vi "Dashboard Main.vi"() -> ()   [LabVIEW 2019]
uses:
  2021-MARS-Swerve/Subsystems/Drive/Drive_Orientation_States.ctl
  <vilib>/Utility/miscctls.llb/LVRowAndColumnTypeDef.ctl
  <vilib>/event_ctls.llb/eventvkey.ctl
  77231be5-4dfd-47d5-a2ff-3724d3268e1c.vi
  6c3be22e-c06e-40dd-b218-0ec3cd26438d.vi
  2be0e37a-cf1f-4fec-827e-dc22e69ce85b.vi
  b3ffd77c-c7a0-4f90-8868-8b56e10d7f8c.vi
  67fa5a46-adf3-4589-a2f7-66a250c43ad7.vi
  788908d1-300c-4db3-916d-f2facaeaae96.vi
  e87f41cb-5a92-4aba-b85e-f5fa50e1b7bd.vi
  bca209f3-dc8a-45d9-88b4-0d3b0861506d.vi
  fb4473b5-3a86-49a6-a9b5-0e1129129e81.vi
  849cc23d-0ef3-4264-9ef7-306e991d33d4.vi
  16c4a620-4255-445b-bb5a-a821105b922f.vi
  55761e46-cf36-4bf9-9854-b902932db1d3.vi
  <vilib>/Rock Robotics/Network Tables/NT Write Boolean.vi
  <vilib>/Rock Robotics/Network Tables/NT Read Boolean.vi
  MARS Created VIs/GlobalDataNames.vi
  <vilib>/Rock Robotics/Network Tables/NT Read Boolean Array.vi
  <vilib>/Rock Robotics/Network Tables/NT Read Numeric Array.vi
  <vilib>/Rock Robotics/Network Tables/NT Write Boolean Array.vi
  <vilib>/Rock Robotics/Network Tables/NT Write String Array.vi
  <vilib>/Rock Robotics/Network Tables/NT Write Numeric Array.vi
  <vilib>/Rock Robotics/WPI/Dashboard/WPI_DashboardLogging Global.vi
  <vilib>/Utility/Data Type/NI_Data Type.lvlib
  <vilib>/Utility/Data Type/Type Definitions/Data Type.ctl
panel:
  in  "Rec Mode":enum32{"Stop", "Record", "Playback"}(radio)
  in  "Camera Name Right":string(combo)="No Camera Selection"
  in  "Camera Settings Right":T1={"Frame Rate"=15, "Compression"=30, "Size"=1, "DB Camera Config"=FALSE} {"Frame Rate" scale=1.0..30.0; "Compression" scale=100.0..-1.0; "Size" items=["640x480", "320x240", "160x120"]}
  out "Driver Controls":string="pilot-\nleft joystick X & Y axes- strafe / lateral and vertical throttle\nright joystick X axis- rotational throttle\nX button- toggle between robot- and field-oriented control modes\nright bumper- auto-target\nLB- outtake\nLT- intake (toggle)\nRT- fire + flywheel spin-up\nA- Zero Drive IMU\nD-pad North: Manual Magazine Forward\nD-pad South: Manual Magazine Backward\nView Button (Left): Manual Cowl Up\nMenu Button (Right): Manual Cowl Down\n\ncopilot-\nright joystick X axis- manual turret control\nX button: Zero Turret Spin\n"
  in  "TCP":refnum<k5>
  out "Robot IP":string="0.0.0.0"
  out "Image Message":string="Timeout in Camera Communications"
  in  "Dashboard Tab":T2(tab)=enum."Operation"
  in  "Max_Ground_Speed(ft/s)":dbl
  in  "Cowl_Kp":dbl=0.06
  in  "Manual_Magazine_Power":dbl=0.4
  in  "Magazine_Firing_Throttle":dbl=0.6
  in  "Intake_Speed (%vbus)":dbl=1.0
  in  "Flywheel_Speed_Multiplier":dbl=1.0
  in  "Flywheel_Acceptable_Error":dbl=200.0
  in  "Turret_Upper_Limit":dbl=160.0
  in  "Turret_Lower_Limit":dbl=-160.0
  in  "Turret_Kd":dbl=0.001
  in  "Turret_Ki":dbl=1e-05
  in  "Turret_Kp":dbl=0.06
  in  "BL_Min Output":dbl=-0.5 min=0.0
  in  "BR_Max Ouput":dbl=0.5 min=0.0
  in  "BR_Int Error Window":dbl=20.0 min=0.0
  in  "BR_N-Int":i32=10 min=0
  in  "BR_N-Diff":i32=10 min=0
  in  "BR_Kd":dbl min=0.0
  in  "BR_Ki":dbl min=0.0
  in  "BR_Kp":dbl=0.0028 min=0.0
  in  "BL_Min Output":dbl=-0.5 min=0.0
  in  "BL_Max Ouput":dbl=0.5 min=0.0
  in  "BL_Int Error Window":dbl=20.0 min=0.0
  in  "BL_N-Int":i32=10 min=0
  in  "BL_N-Diff":i32=10 min=0
  in  "BL_Kd":dbl min=0.0
  in  "BL_Ki":dbl min=0.0
  in  "BL_Kp":dbl=0.0028 min=0.0
  in  "FL_Min Output":dbl=-0.5 min=0.0
  in  "FL_Max Ouput":dbl=0.5 min=0.0
  in  "FL_Int Error Window":dbl=20.0 min=0.0
  in  "FL_N-Int":i32=10 caption="FR_N-Int" min=0
  in  "FL_N-Diff":i32=10 min=0
  in  "FL_Kd":dbl min=0.0
  in  "FL_Ki":dbl min=0.0
  in  "FL_Kp":dbl=0.0028 min=0.0
  in  "FR_Min Output":dbl=-0.5 min=0.0
  in  "FR_Max Ouput":dbl=0.5 min=0.0
  in  "FR_Int Error Window":dbl=20.0 min=0.0
  in  "FR_N-Int":i32=10 min=0
  in  "FR_N-Diff":i32=10 min=0
  in  "FR_Kd":dbl min=0.0
  in  "FR_Ki":dbl min=0.0
  in  "FR_Kp":dbl=0.0028 min=0.0
  in  "Auto_Play_Selector":string(combo)="Play 1"
  out "Cowl_Position(Degrees)":dbl(knob)=45.0 scale=-180.0..180.0
  out "Flywheel_Spun_Up":bool
  out "Turret_Auto_Targetted":bool
  out "Orientation_State":T3
  out "Back_Right_Drive_Command":dbl(slide) scale=0.0..1.0 scale format="%.2f"
  out "Back_Right_Angle_Command(deg)":dbl(knob) scale=180.0..-180.0 scale format="%#_6f"
  out "Back_Left_Drive_Command":dbl(slide) scale=0.0..1.0 scale format="%.2f"
  out "Back_Left_Angle_Command(deg)":dbl(knob) scale=180.0..-180.0 scale format="%#_6f"
  out "Front_Left_Drive_Command":dbl(slide) scale=0.0..1.0 scale format="%.2f"
  out "Front_Left_Angle_Command(deg)":dbl(knob) scale=180.0..-180.0 scale format="%#_6f"
  out "Front_Right_Drive_Command":dbl(slide) scale=0.0..1.0 scale format="%.2f"
  out "Front_Right_Angle_Command(deg)":dbl(knob) scale=180.0..-180.0 scale format="%#_6f"
  out "Flywheel_Velocity(RPM)":dbl(slide)=2614.0 scale=0.0..5000.0 scale format="%#_5g"
  out "Turret_Absolute_Position(Degrees)":dbl(knob)=45.0 scale=-180.0..180.0
  out "Camera Image":T4(plugin-control)
  in  "Camera Name":string(combo)="No Camera Selection"
  in  "Camera Settings":T1={"Frame Rate"=15, "Compression"=30, "Size"=1, "DB Camera Config"=TRUE} {"Frame Rate" scale=1.0..30.0; "Compression" scale=100.0..-1.0; "Size" items=["640x480", "320x240", "160x120"]}
  out "Camera Perf":string="                          "
  out "BoolTableSize":i32
  out "NumTableSize":i32
  out "StrTableSize":i32
  out "Selector":string="Initialize"
  out "NTEmpty":bool=TRUE
  out "disconnected":bool=TRUE
  out "ValuesGotOverwritten":bool
  in  "Select Auto":string(combo)="Select Autonomous ..."
  out "NT Connection":bool
  out "JS1 Z":dbl(slide) scale=-1.0..1.0 scale format="%#_2e"
  out "JS1 Graph":cluster{"X":dbl, "Y":dbl}[](graph)
  out "JS1 Buttons":T5
  out "JS2 Z":dbl(slide) scale=-1.0..1.0 scale format="%#_2e"
  out "JS2 Graph":cluster{"X":dbl, "Y":dbl}[](graph)
  out "JS2 Buttons":T5
  out "Mode":T6(ring)=enum."Disconnected"
  out "Right Camera Perf":cluster{"Bandwidth (Mbps)":dbl, "FPS":dbl}
  out "Camera Image Right":T4(plugin-control)
  in  "DB/String 9":string
  in  "DB/String 8":string
  in  "DB/String 7":string
  in  "DB/String 6":string
  in  "DB/String 5":string
  in  "DB/String 4":string
  in  "DB/String 3":string
  in  "DB/String 2":string
  in  "DB/String 1":string
  in  "DB/String 0":string
  in  "DB/Slider 0":dbl(slide) scale=0.0..5.0
  in  "DB/Slider 1":dbl(slide) scale=0.0..5.0
  in  "DB/Slider 2":dbl(slide) scale=0.0..5.0
  in  "DB/Slider 3":dbl(slide) scale=0.0..5.0
  out "DB/LED 3":bool
  out "DB/LED 2":bool
  out "DB/LED 1":bool
  out "DB/LED 0":bool
  in  "DB/Button 3":bool
  in  "DB/Button 2":bool
  in  "DB/Button 1":bool
  in  "DB/Button 0":bool caption="New Name"
  in  "Test Slider":dbl(slide) scale=0.0..100.0 scale format="%#_3g"
  in  "On/Off":bool caption="Solenoid"
  in  "Test Name":u16(ring) items=["Select the test to run..."]
  in  "Test Tree":string(tree)
  in  "Motor":cluster{"Value":dbl, "Enable":bool} {"Value" scale=-1.0..1.0 scale format="%#_3g"}
  out "Progress":T7 {"Test Progress" scale=0.0..100.0}
  in  "Rev/Fwd":cluster{"Forward":bool, "Reverse":bool}
  in  "Test Ring":u16(ring) items=["Monochrome", "Color"]
  out "Cmd Status":string
  in  "Execute Command":bool
  in  "Command Params":string[][](table)
  in  "Command Selection":i32(listbox)
  in  "CheckList":i32(listbox)
  out "Tree":string(tree)
  out "Background":bool
  # "HW"
  # "Cowl"
  # "Constant"
  # "Turret"
  # "Flywheel"
  # "Intake"
  # "Drive"
  # "Magazine"
  # "Drive Commands"
  # "Front_Left"
  # "Front_Right"
  # "Back_Left"
  # "Back_Right"
  # "HW"
  # "Joysticks"
  # "Drive Motors"
  # "Front"
  # "Right"
  # "Left"
  # "Back"
  # "This tab is a great place for autonomous settings and robot-specific values.\nPlace controls and indicators inside this tab and match name to\nDashboard Variables on robot. You can also delete this comment."
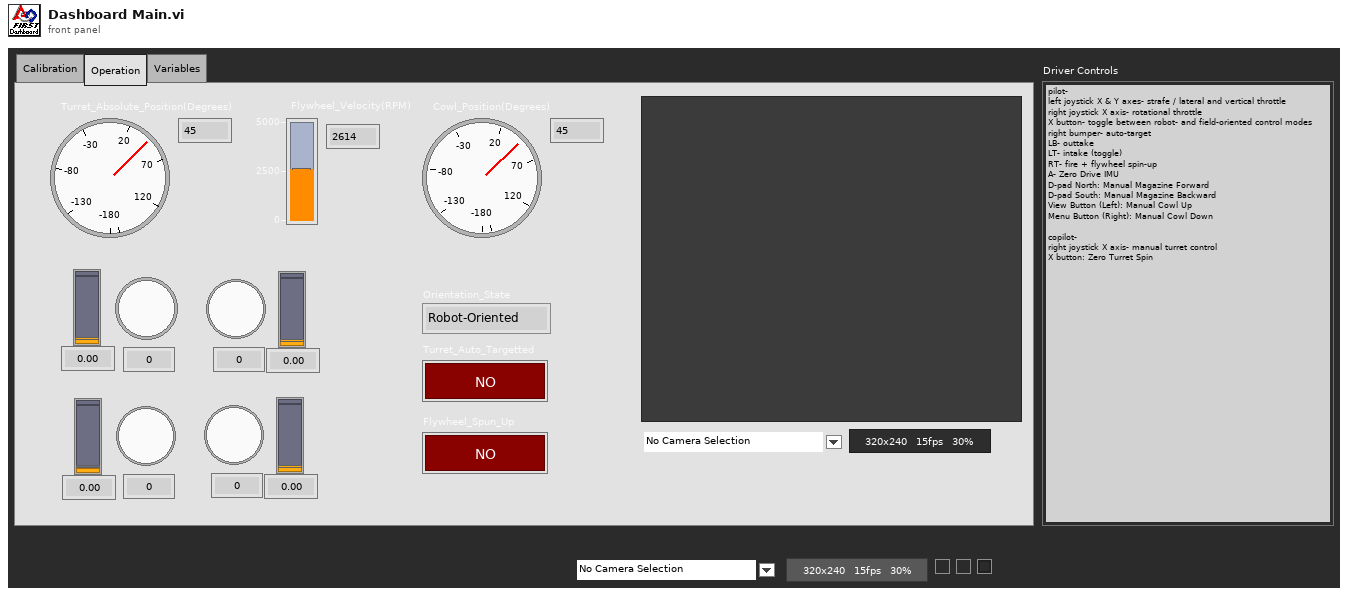
[diagram p1: front panel]
types:
  T1 = cluster{"Frame Rate":i32, "Compression":i32, "Size":u16, "DB Camera Config":bool}
  T2 = enum32{"Calibration", "Operation", "Testing", "Drive", "Camera", "Basic", "Custom", "Test", "Commands", "Checklist", "Variables"}
  T3 = typedef "Drive_Orientation_States.ctl" = enum16{"Robot-Oriented", "Field-Oriented"}
  T4 = typedef "IMAQ Image.ctl" = refnum<image>
  T5 = cluster{bool, bool, bool, bool, bool, bool, bool, bool, bool, bool, bool, bool}
  T6 = enum8{"Tele-Op Disabled", "Tele-Op Enabled", "Auto Disabled", "Auto Enabled", "Test Disabled", "Test Enabled", "Disconnected", "No Code", "E-Stop"}
  T7 = cluster{"Test Progress":u8, "Test Progress Text":string}
  T8 = cluster{"Save Path":path, "Interval (s)":dbl, "Keep":i32}
  T9 = enum32{"Drive", "Camera", "Basic", "Custom", "Test", "Commands", "Checklist", "Variables"}
  T10 = typedef "Image Type" = u32
  T11 = cluster{"IDs":cluster{"RPC field ID":u16, "Unique ID":u16}, "String":string}
  T12 = cluster{"Error Strings":string, "Disable Counts":cluster{u16, u16}, "Rail Faults":cluster{u16, u16, u16}, "Robot IP":string, "DB Mode":u8, "Event Info":cluster{"Name":string, "Type":u8, "Number":u16, "Replay":u8}}
  T13 = cluster{"Storage":cluster{"Disk Free":u64, "RAM Block":u32, "RAM free":u32}, "CPU Utilization":cluster{"CPU % ISR":sgl, "CPU % Time Crit":sgl, "CPU % Timed Str":sgl, "CPU % High":sgl, "CPU % Above":sgl, "CPU % Normal":sgl, "CPU % Low":sgl}, "CAN":cluster{"% Bus Utilization":sgl, "Bus Off Cnt":u32, "TX_FIFO Full Cnt":u32, "Receive Error Cnt":u8, "Transmit Error Cnt":u8}, "HID":cluster{"HID Outputs":u32, "Rumble Low":u16, "Rumble High":u16}[]}
  T14 = cluster{"Status bits":cluster{"Test Mode":bool, "Autonomous":bool, "Enabled":bool, "Code Start":bool, "Brownout":bool, "Reserved 2":bool, "Reserved 3":bool, "E-Stop":bool}, "Code Trace":cluster{"Disabled":bool, "TeleOp":bool, "Auto":bool, "Test":bool}, "Controller Type":enum16{"unknown", "cRIO", "roboRio"}, "Code?":enum16{"unknown", "noCode", "code"}, "Battery V":dbl}
  T15 = cluster{"Control Bits":cluster{"TestMode":bool, "Autonomous":bool, "Enabled":bool, "FMS Present":bool, bool, bool, bool, "E-Stop":bool}, "Team Station ":u8, "Countdown":sgl, "Joystick Values":cluster{"Axes":dbl[], "Buttons":bool[], "POVs":i16[]}[]}
  T16 = cluster{"Axes":dbl[], "Buttons":bool[], "POVs":i16[]}[]
  T17 = cluster{"Axes":dbl[], "Buttons":bool[], "POVs":i16[]}
  T18 = cluster{"Buttons[0]":bool, "Buttons[1]":bool, "Buttons[2]":bool, "Buttons[3]":bool, "Buttons[4]":bool, "Buttons[5]":bool, "Buttons[6]":bool, "Buttons[7]":bool, "Buttons[8]":bool, "Buttons[9]":bool, "Buttons[10]":bool, "Buttons[11]":bool}
  T19 = cluster{"Camera Image":refnum<vi>, "Dashboard Tab":refnum<vi>, "Background":refnum<vi>, "Rec Mode":refnum<vi>, "Test Slider":refnum<vi>, "On/Off ":refnum<vi>, "Test Ring":refnum<vi>, "Rev/Fwd":refnum<vi>, "Test Name":refnum<vi>, "Motor":refnum<vi>, "Progress":refnum<vi>, "CheckList":refnum<vi>, "Tree":refnum<vi>, "Test Tree":refnum<vi>, "Command Params":refnum<vi>, "Command Selection":refnum<vi>, "Execute Command":refnum<vi>, "Cmd Status":refnum<vi>, "Camera Settings":refnum<vi>, "Camera Name":refnum<vi>, "Camera Perf":refnum<vi>, "Camera Settings Right":refnum<vi>, "Camera Name Right":refnum<vi>, "Camera Image Right":refnum<vi>}
  T20 = cluster{"Global Rectangle":i32[], "Contours":cluster{"Contour Type":u32, "ROI Type":u32, "Points":i32[]}[]}
  T21 = cluster{"Camera Name":string, string, "Saved DB Images Info":cluster{"Save Path":path, "Interval (s)":dbl, "Keep":i32}}
  T22 = cluster{"Camera Name Right":string, string, "Saved DB Images Info":cluster{"Save Path":path, "Interval (s)":dbl, "Keep":i32}}
  T23 = cluster{"Operation":enum16{"Update", "Clear"}, "Color Box":u32}[]
  T24 = typedef "eventvkey.ctl" = enum16{"ASCII", "Enter", "Return", "Shift", "Ctrl", "Alt", "Cmd", "Opt", "Caps", "NumLock", "Clear", "Break", "Up", "Down", "Left", "Right", "Insert", "Delete", "Home", "End", "PageUp", "PageDown", "Escape", "Help", "Pause", "ScrollLock", "F1", "F2", "F3", "F4", "F5", "F6", "F7", "F8", "F9", "F10", "F11", "F12", "F13", "F14", "F15", "F16", "F17", "F18", "F19", "F20", "F21", "F22", "F23", "F24", "Play", "VolumeUp", "VolumeDown", "Mute", "Two Byte Char"}
  T25 = cluster{"Image Size":bool, "Image Type":bool, "Pixel Value":bool, "ROI Information":bool, "Zoom Factor":bool}
  T26 = cluster{"Operation":enum16{"Update", "Clear"}, "Color Box":u32}
  T27 = typedef "LVRowAndColumnTypeDef.ctl" = cluster{"Row":i32, "Column":i32}
  T28 = cluster{"Shift":bool, "Ctrl":bool, "Alt":bool, "Cmd":bool, "Opt":bool}
  T29 = typedef "NI_Data Type.lvlib/Data Type.ctl" = enum8{"Invalid Type", "Void", "I8", "I16", "I32", "I64", "U8", "U16", "U32", "U64", "Single Float", "Double Float", "Extended Float", "Single Complex", "Double Complex", "Extended Complex", "Enum U8", "Enum U16", "Enum U32", "Enum U64", "Single Float With Unit", "Double Float With Unit", "Extended Float With Unit", "Single Complex with Unit", "Double Complex with Unit", "Extended Complex with Unit", "Boolean", "String", "Path", "Picture", "Tag", "Array", "Cluster", "Variant", "LV Variant", "Waveform", "Timestamp", "Digital Waveform", "Digital Data", "ExpressData", "Refnum", "External Data", "VI", "Poly VI", "LabVIEW Class Instance", "Fixed Point", "Set Collection", "Map Collection"}
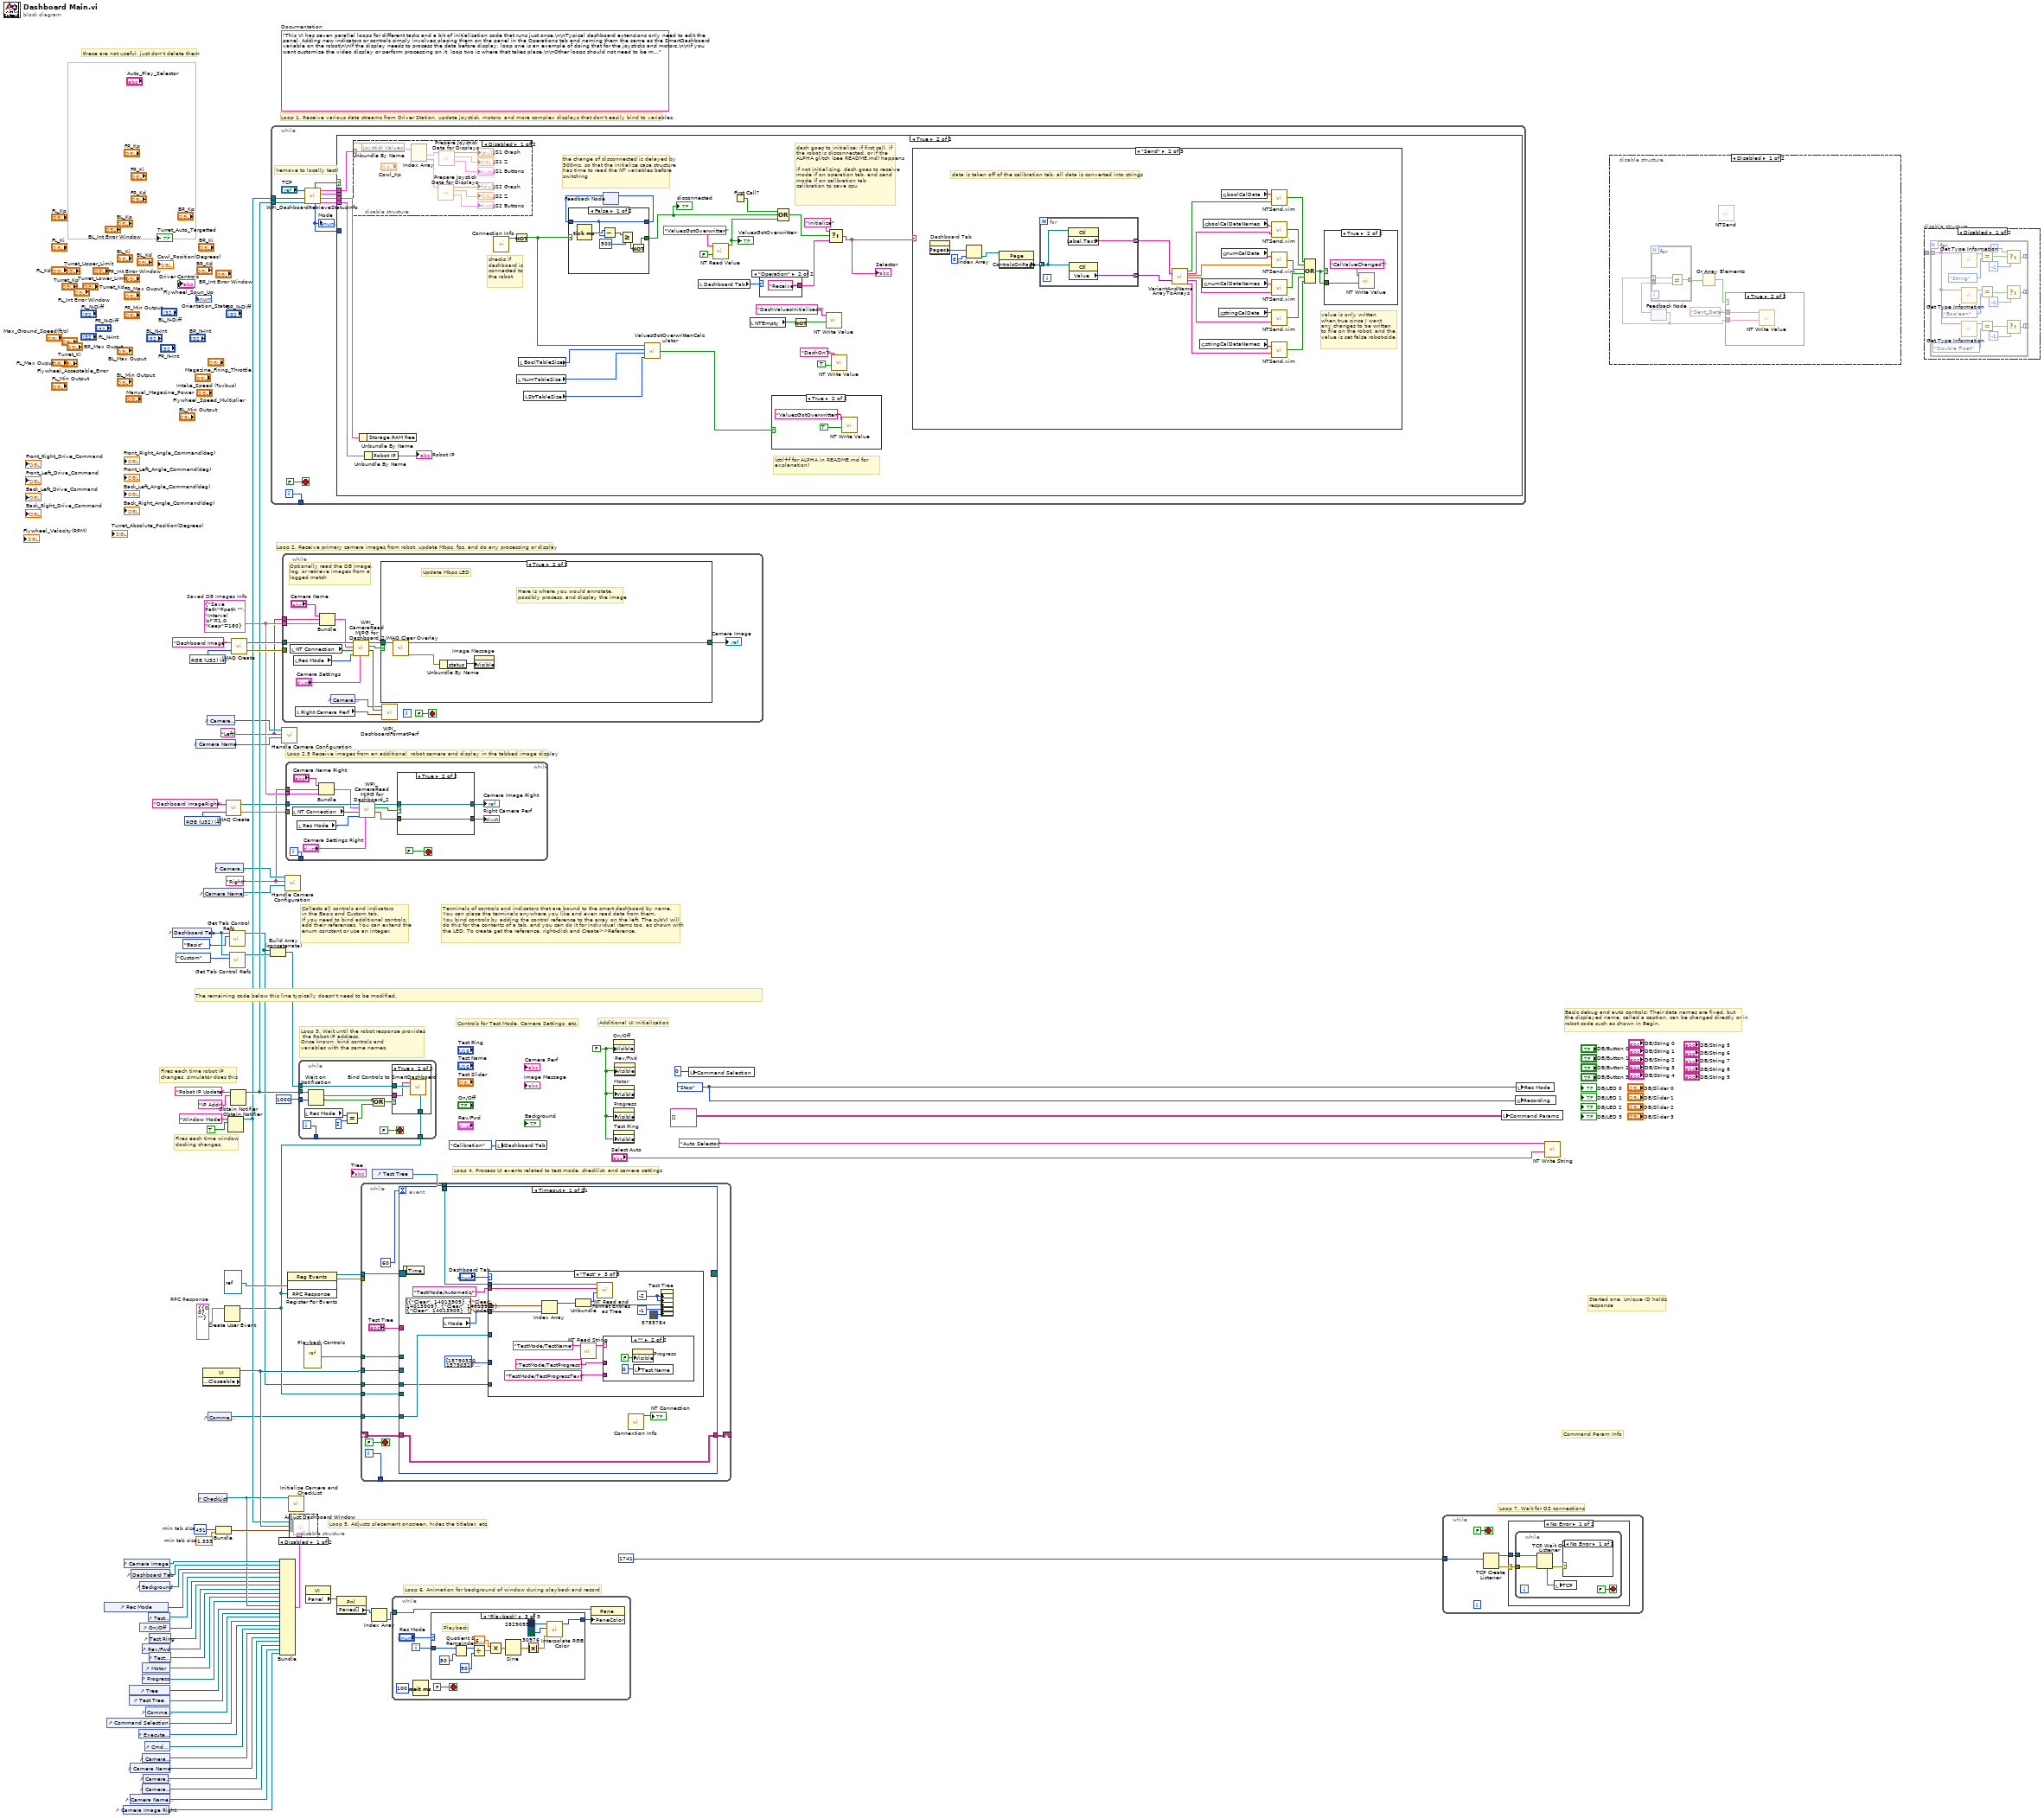
[diagram p0: block diagram]
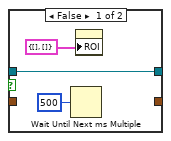
[diagram p6: hidden frame]
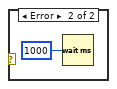
[diagram p7: hidden frame]
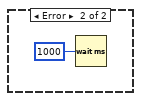
[diagram p8: hidden frame]
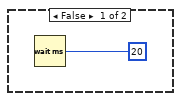
[diagram p9: hidden frame]
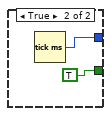
[diagram p11: hidden frame]
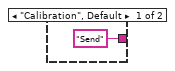
[diagram p13: hidden frame]
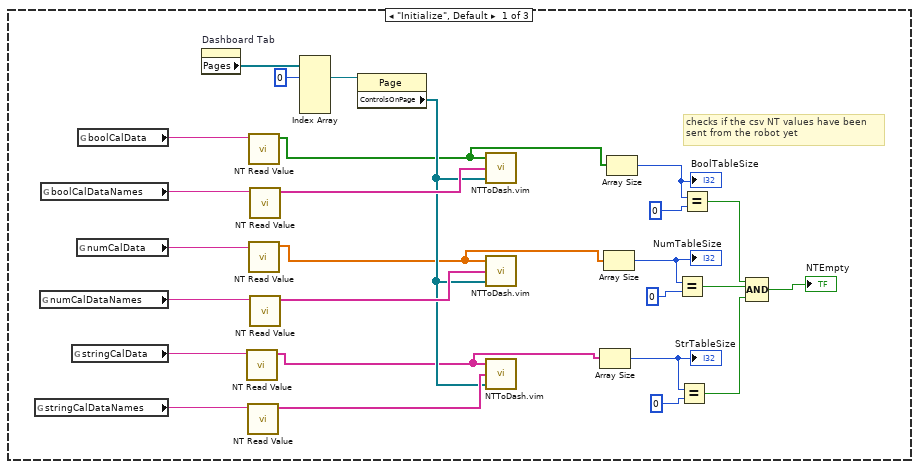
[diagram p14: hidden frame]
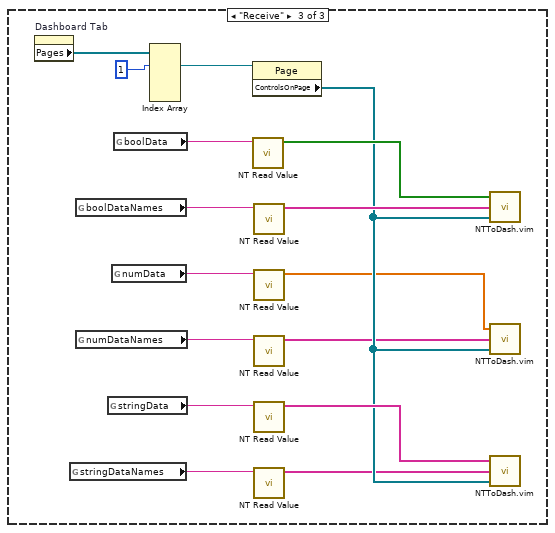
[diagram p16: hidden frame]
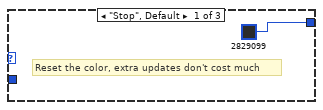
[diagram p17: hidden frame]
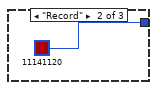
[diagram p18: hidden frame]
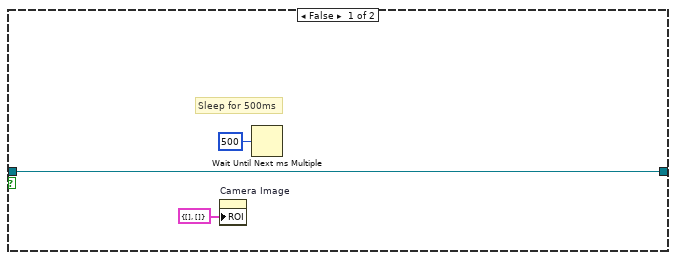
[diagram p20: hidden frame]
diagram:
  w4 = T8 {"Save Path"=path "", "Interval (s)"=1.0, "Keep"=180}  # Saved DB Images Info
  w3 = "Right"
  w2 = "Left"
  w14 = T10 4 items=["Grayscale (U8)", "Grayscale (I16)", "Grayscale (SGL)", "Complex (CSG)", "RGB (U32)", "HSL (U32)", "RGB (U64)"] ("Image Type")
  w30 = T11 {"IDs"={"RPC field ID"=0, "Unique ID"=0}, "String"=""}  # RPC Response
  w52 = 491  # min tab size
  w51 = 1.333  # min tab size
  w59 = enum32{"Stop", "Record", "Playback"}."Stop" ("Rec Mode")
  w36 = FALSE ("Visible")
  (unwired) "This VI has seven parallel loops for different tasks and a bit of initialization code that runs just once.\n\nTypical dashboard extensions only need to edit the panel. Adding new indicators or controls simply involves placing them on the panel in the Operations tab and naming them the same as the SmartDashboard variable on the robot\n\nIf the display needs to process the data before display, loop one is an example of doing that for the joysticks and motors.\n\nIf you want customize the video display or perform processing on it, loop two is where that takes place.\n\nOther loops should not need to be modified. They are pretty standard, and document the task they perform."  # Documentation
  w76 = T10 4 items=["Grayscale (U8)", "Grayscale (I16)", "Grayscale (SGL)", "Complex (CSG)", "RGB (U32)", "HSL (U32)", "RGB (U64)"] ("Image Type")
  # "these are not useful, just don't delete them"
  # "Loop 2.5 Receive images from an additional  robot camera and display in the tabbed image display"
  # "Command Param Info"
  # "Started one, Unique ID holds\nresponse"
  # "Loop 7. Wait for DS connections"
  # "Basic debug and auto controls: Their data names are fixed, but\nthe displayed name, called a caption, can be changed directly or in\nrobot code such as shown in Begin."
  # "Controls for Test Mode, Camera Settings, etc."
  # "Additional UI Initialization"
  # "Loop 6. Animation for background of window during playback and record"
  # "Fires each time robot IP\nchanges, simulator does this"
  # "Fires each time window\ndocking changes."
  # "Collects all controls and indicators\nin the Basic and Custom tab.\nIf you need to bind additional controls,\nadd their references. You can extend the\nenum constant or use an integer."
  # "The remaining code below this line typically doesn't need to be modified."
  # "Loop 4. Process UI events related to test mode, checklist, and camera settings"
  # "Terminals of controls and indicators that are bound to the smart dashboard by name.\nYou can place the terminals anywhere you like and even read data from them.\nYou bind controls by adding the control reference to the array on the left. The subVI will\ndo this for the contents of a tab, and you can do it for individual items too, as shown with\nthe LED. To create get the reference, right-click and Create>>Reference."
  # "Loop 3. Wait until the robot response provides\n the Robot IP address.\nOnce known, bind controls and\nvariables with the same names."
  # "Loop 5. Adjusts placement onscreen, hides the titlebar, etc."
  # "Loop 1. Receive various data streams from Driver Station, update joystick, motors, and more complex displays that don't easily bind to variables."
  # "Loop 2. Receive primary camera images from robot, update Mbps, fps, and do any processing or display"
  n1 = control-ref of="Rec Mode"() -> (w42:refnum<vi>)
  n2 = control-ref of="Command Selection"() -> (w29:refnum<vi>)
  n3 = control-ref of="Camera Image Right"() -> (w7:refnum<vi>)
  n4 = control-ref of="Camera Image"() -> (w54:refnum<vi>)
  n5 = control-ref of="Tree"() -> (w46:refnum<vi>)
  n6 = control-ref of="Test Tree"() -> (w45:refnum<vi>)
  n7 = control-ref of="Camera Name"() -> (w20:refnum<vi>)
  n8 = control-ref of="Camera Name Right"() -> (w8:refnum<vi>)
  n9 = control-ref of="Dashboard Tab"() -> (w53:refnum<vi>)
  n10 = control-ref of="Execute Command"() -> (w31:refnum<vi>)
  n11 = control-ref of="Background"() -> (w49:refnum<vi>)
  n12 = control-ref of="On/Off"() -> (w40:refnum<vi>)
  n13 = control-ref of="Progress"() -> (w37:refnum<vi>)
  n14 = control-ref of="Camera Settings"() -> (w21:refnum<vi>)
  n15 = control-ref of="Camera Settings Right"() -> (w9:refnum<vi>)
  n16 = control-ref of="Rev/Fwd"() -> (w38:refnum<vi>)
  n17 = control-ref of="Motor"() -> (w43:refnum<vi>)
  n18 = control-ref of="Camera Perf"() -> (w19:refnum<vi>)
  n19 = control-ref of="Cmd Status"() -> (w25:refnum<vi>)
  n20 = control-ref of="Command Params"() -> (w32:refnum<vi>)
  n21 = control-ref of="Test Slider"() -> (w41:refnum<vi>)
  n22 = control-ref of="Test Ring"() -> (w39:refnum<vi>)
  n23 = control-ref of="Test Name"() -> (w44:refnum<vi>)
  n24 = control-ref of="Dashboard Tab"() -> (w57:refnum<vi>)
  n25 = control-ref of="Camera Name"() -> (w22:refnum<vi>)
  n26 = control-ref of="CheckList"() -> (w47:refnum<vi>)
  n27 = property class="VI" props=["Front Panel.Closeable"]() -> (reference out=w58:refnum<vi>)  [unwired: 2 in, 2 out]
  n28 = control-ref of="Camera Name Right"() -> (w10:refnum<vi>)
  n29 = control-ref of="Camera Settings"() -> (w23:refnum<vi>)
  n30 = control-ref of="Command Params"() -> (w24:refnum<vi>)
  n31 = control-ref of="Camera Settings Right"() -> (w11:refnum<vi>)
  n32 = Bundle("min tab size"=w52, "min tab size"=w51) -> (w50:cluster{"min tab size":i32, "min tab size":dbl})  [unwired: 1 in]
  n33 = Create User Event(user event datatype=w30) -> (user event=w26:refnum<user-event>)  [unwired: 1 in, 1 out]
  n34 = call "IMAQ Create"("Image Name"="Dashboard ImageRight", "Image Type"=w14) -> ("New Image"=w13:T4, "error out"=w12:errorcluster)  [unwired: 2 in, 1 out]
  n35 = Obtain Notifier(name (unnamed)="Window Mode", notification data type=TRUE) -> (notifier out=w34:refnum<notifier>)  [unwired: 2 in, 2 out]
  n36 = call <vilib>:"Get Tab Control Refs.vi"("Page Index"=T9."Basic" ("Dashboard Tab"), "TabControl in"=w57) -> ("ControlsOnPage"=w18:refnum<vi>[])  [unwired: 9 in]
  n37 = call <vilib>:"Get Tab Control Refs.vi"("Page Index"=T9."Custom" ("Dashboard Tab"), "TabControl in"=w57) -> ("ControlsOnPage"=w56:refnum<vi>[])  [unwired: 9 in]
  n38 = Obtain Notifier(name (unnamed)="Robot IP Update", notification data type="IP Addr" ("name (unnamed)")) -> (notifier out=w35:refnum<notifier>)  [unwired: 2 in, 2 out]
  n39 = call "IMAQ Create"("Image Name"="Dashboard Image", "Image Type"=w76) -> ("New Image"=w74:T4, "error out"=w73:errorcluster)  [unwired: 2 in, 1 out]
  n40 = Build Array (concatenate)(w18, w56) -> (w55:refnum<vi>[])
  n41 = while {
    tunnel: [w86] -> _
    tunnel: w35 -> [w81]
    tunnel: w34 -> [w78]
    i -> [w86]
    stop <- FALSE stop-if-true
    # "(remove to locally test)"
    n42 = call <vilib>:"WPI_DashboardRetrieveStatusInfo.vi"("Binding Refnum"=w81, "Window Mode Notifier"=w78, "TCP Cnx"="TCP") -> ("Power and Errors"=w82:T12, "Robot Metrics"=w84:T13, "Status Info"=w85:T14, "Control Info"=w83:T15, "Robot Mode"=w80:T6, "Process?"=w77:bool)  [unwired: 3 in]
    "Mode" <- w80
    n43 = case shown="True" w77 {
      tunnel: w85 -> [_ _]
      tunnel: w84 -> [_ w115]
      tunnel: w83 -> [_ w114]
      tunnel: w82 -> [_ w113]
      tunnel: w80 -> [_ _]
      frame False {
        n44 = Wait (ms)(milliseconds to wait=u32 20) -> ()  [unwired: 1 out]
      }
      frame True {
        # "checks if dashboard is connected to the robot"
        # "(ctrl+f for ALPHA in README.md for explanation)"
        # "the change of disconnected is delayed by 500ms, so that the initialize case structure has time to read the NT variables before switching"
        # "dash goes to initialize: if first call, if\nthe robot is disconnected, or if the ALPHA glitch (see README.md) happens\n\nif not initializing, dash goes to receive mode if on operation tab, and send mode if on calibration tab\ncalibration to save cpu"
        n45 = disable-structure shown="Disabled" {
          disable-tunnel: w114 -> [w135 _]
          frame Disabled {
            n46 = Unbundle By Name(w135) -> ("Joystick Values"=w134:T16)
            n47 = Index Array(array=w134) -> (element #1=w133:T17, element #2=w129:T17)  [unwired: 2 in]
            n48 = call "Prepare Joystick Data for Displays.vi"("Joystick Values"=w129) -> ("Buttons"=→"JS2 Buttons":T18, "Z Axis"=→"JS2 Z":dbl, "Cartesian Data"=→"JS2 Graph":cluster{"X axis":dbl, "X axis":dbl}[])  [unwired: 8 in]
            n49 = call "Prepare Joystick Data for Displays.vi"("Joystick Values"=w133) -> ("Buttons"=→"JS1 Buttons":T18, "Z Axis"=→"JS1 Z":dbl, "Cartesian Data"=→"JS1 Graph":cluster{"X axis":dbl, "X axis":dbl}[])  [unwired: 8 in]
          }
          frame Enabled {
          }
        }
        n50 = Unbundle By Name(w115) -> ()  [unwired: 1 out]
        n51 = Unbundle By Name(w113) -> ("Robot IP"=→"Robot IP":string)
        n52 = call <vilib>:"Connection Info.vi"() -> ("Connected"=w101:bool)  [unwired: 10 in, 1 out]
        n53 = Not(x=w101) -> (.not. x?=w94:bool)
        n54 = local read "NumTableSize"() -> (w96:i32)
        n55 = local read "BoolTableSize"() -> (w97:i32)
        n56 = local read "StrTableSize"() -> (w95:i32)
        n57 = feedback #1() -> (w98:u32)  [unwired: 1 in]
        n58 = case shown="False" w94 {
          tunnel: [w118 TRUE] -> w100
          tunnel: [w122 w124] -> w99
          tunnel: w98 -> [w122 _]
          frame False {
            n59 = Tick Count (ms)() -> (millisecond timer value=w123:u32)
            n60 = Subtract(x=w123, y=w122) -> (x-y=w121:u32)
            n61 = Greater Or Equal?(x=w121, y=u32 500) -> (x >= y?=w119:bool)
            n62 = Not(x=w119) -> (.not. x?=w118:bool)
          }
          frame True {
            n63 = Tick Count (ms)() -> (millisecond timer value=w124:u32)
          }
        }
        "disconnected" <- w100
        n64 = feedback-in #1(w99) -> ()
        n65 = call "ValuesGotOverwrittenCalculator.vi"("StrTableSize"=w95, "NumTableSize"=w96, "BoolTableSize"=w97, "disconnected"=w94) -> ("ValuesGotOverwritten"=w93:bool)
        n66 = local read "Dashboard Tab"() -> (w109:T2)
        n67 = call-poly <vilib>:"NT Read Value.vi"("Default Value"=FALSE, "Name"="ValuesGotOverwritten") -> ("Boolean"=w90:bool)  [unwired: 8 in, 1 out]
        "ValuesGotOverwritten" <- w90
        n68 = First Call?() -> (First Call?: T/F=w102:bool)
        n69 = local read "NTEmpty"() -> (w104:bool)
        n70 = case shown="\"Operation\"" w109 {
          tunnel: ["Send" "Receive"] -> w108
          frame "Calibration", Default {
          }
          frame "Operation" {
          }
        }
        n71 = case shown="True" w93 {
          frame False {
          }
          frame True {
            n72 = call-poly <vilib>:"NT Write Value.vi"("Boolean"=TRUE, "Name"="ValuesGotOverwritten") -> ()  [unwired: 9 in, 1 out]
          }
        }
        n73 = Compound Arithmetic op=OR(w102, w100, w90) -> (w106:bool)
        n74 = Not(x=w104) -> (.not. x?=w103:bool)
        n75 = call-poly <vilib>:"NT Write Value.vi"("Boolean"=w103, "Name"="DashValuesInitialized?") -> ()  [unwired: 9 in, 1 out]
        n76 = Select(t="Initialize", s=w106, f=w108) -> (s? t:f=w89:string)
        "Selector" <- w89
        n77 = call-poly <vilib>:"NT Write Value.vi"("Boolean"=TRUE, "Name"="DashOn?") -> ()  [unwired: 9 in, 1 out]
        n78 = case shown="\"Send\"" w89 {
          frame "Initialize", Default {
            # "checks if the csv NT values have been\nsent from the robot yet"
            n79 = global read "GlobalDataNames.vi" "stringCalDataNames"() -> (w151:string)
            n80 = global read "GlobalDataNames.vi" "numCalDataNames"() -> (w153:string)
            n81 = global read "GlobalDataNames.vi" "boolCalDataNames"() -> (w156:string)
            n82 = global read "GlobalDataNames.vi" "stringCalData"() -> (w152:string)
            n83 = global read "GlobalDataNames.vi" "numCalData"() -> (w154:string)
            n84 = global read "GlobalDataNames.vi" "boolCalData"() -> (w155:string)
            n85 = property on="Dashboard Tab" class="TabCtl (strict)"() -> ("Pages"=w157:refnum<vi>[])  [unwired: 2 in, 2 out]
            n86 = call-poly <vilib>:"NT Read Value.vi"("Name"=w152) -> ("String Array"=w148:string[])  [unwired: 9 in, 1 out]
            n87 = call-poly <vilib>:"NT Read Value.vi"("Name"=w151) -> ("String Array"=w162:string[])  [unwired: 9 in, 1 out]
            n88 = call-poly <vilib>:"NT Read Value.vi"("Name"=w155) -> ("Boolean Array"=w150:bool[])  [unwired: 9 in, 1 out]
            n89 = call-poly <vilib>:"NT Read Value.vi"("Name"=w154) -> ("Numeric Array"=w149:dbl[])  [unwired: 9 in, 1 out]
            n90 = call-poly <vilib>:"NT Read Value.vi"("Name"=w156) -> ("String Array"=w163:string[])  [unwired: 9 in, 1 out]
            n91 = call-poly <vilib>:"NT Read Value.vi"("Name"=w153) -> ("String Array"=w161:string[])  [unwired: 9 in, 1 out]
            n92 = Index Array(array=w157, index #1=0 ("index")) -> (element #1=w160:refnum<vi>)  [unwired: 4 in, 4 out]
            n93 = property class="Page"(reference=w160) -> ("ControlsOnPage"=w158:refnum<vi>[])  [unwired: 1 in, 2 out]
            n94 = call "NTToDash.vim"("Controls on Page[]"=w158, "Names Array"=w163, "Data Array"=w150) -> ()  [unwired: 1 in]
            n95 = call "NTToDash.vim"("Controls on Page[]"=w158, "Names Array"=w161, "Data Array"=w149) -> ()  [unwired: 1 in]
            n96 = call "NTToDash.vim"("Controls on Page[]"=w158, "Names Array"=w162, "Data Array"=w148) -> ()  [unwired: 1 in]
            n97 = Array Size(array=w148) -> (size(s)=w143:i32)
            "StrTableSize" <- w143
            n98 = Array Size(array=w149) -> (size(s)=w145:i32)
            "NumTableSize" <- w145
            n99 = Array Size(array=w150) -> (size(s)=w147:i32)
            "BoolTableSize" <- w147
            n100 = Equal?(x=w145, y=0 ("size(s)")) -> (x = y?=w140:bool)
            n101 = Equal?(x=w143, y=0 ("size(s)")) -> (x = y?=w141:bool)
            n102 = Equal?(x=w147, y=0 ("size(s)")) -> (x = y?=w139:bool)
            n103 = Compound Arithmetic op=AND(w139, w140, w141) -> (→"NTEmpty":bool)
          }
          frame "Send" {
            # "value is only written\nwhen true since I want\nany changes to be written\nto file on the robot, and the \nvalue is set false robot-side"
            # "data is taken off of the calibration tab, all data is converted into strings"
            n104 = property on="Dashboard Tab" class="TabCtl (strict)"() -> ("Pages"=w188:refnum<vi>[])  [unwired: 2 in, 2 out]
            n105 = Index Array(array=w188, index=0) -> (element=w186:refnum<vi>)
            n106 = property class="Page"(reference=w186) -> ("ControlsOnPage"=w185:refnum<vi>[])  [unwired: 1 in, 2 out]
            n107 = for {
              tunnel: w185 -> [w193] mode=indexing
              tunnel: [w192] -> w184 mode=indexing
              tunnel: [w191] -> w183 mode=indexing
              n108 = property class="Ctl"(reference=w193) -> ("Label.Text"=w192:string)  [unwired: 1 in, 2 out]
              n109 = property class="Ctl"(reference=w193) -> ("Value"=w191:variant)  [unwired: 1 in, 2 out]
            }
            n110 = call "VariantAndNameArrayToArrays.vi"("Names Array"=w184, "Variant Array"=w183) -> ("bool"=w182:bool[], "boolNames"=w181:string[], "num"=w179:dbl[], "numNames"=w178:string[], "string"=w164:string[], "stringNames"=w180:string[])  [unwired: 12 in]
            n111 = global read "GlobalDataNames.vi" "stringCalDataNames"() -> (w173:string)
            n112 = global read "GlobalDataNames.vi" "numCalDataNames"() -> (w175:string)
            n113 = global read "GlobalDataNames.vi" "boolCalDataNames"() -> (w176:string)
            n114 = global read "GlobalDataNames.vi" "stringCalData"() -> (w174:string)
            n115 = global read "GlobalDataNames.vi" "numCalData"() -> (w177:string)
            n116 = global read "GlobalDataNames.vi" "boolCalData"() -> (w172:string)
            n117 = call "NTSend.vim"("Array"=w182, "name"=w172) -> ("Write?"=w171:bool)
            n118 = call "NTSend.vim"("Array"=w181, "name"=w176) -> ("Write?"=w170:bool)
            n119 = call "NTSend.vim"("Array"=w179, "name"=w177) -> ("Write?"=w169:bool)
            n120 = call "NTSend.vim"("Array"=w178, "name"=w175) -> ("Write?"=w168:bool)
            n121 = call "NTSend.vim"("Array"=w164, "name"=w174) -> ("Write?"=w167:bool)
            n122 = call "NTSend.vim"("Array"=w180, "name"=w173) -> ("Write?"=w166:bool)
            n123 = Compound Arithmetic op=OR(w171, w170, w169, w168, w167, w166) -> (w165:bool)
            n124 = case shown="True" w165 {
              tunnel: w165 -> [_ w190]
              frame False {
              }
              frame True {
                n125 = call-poly <vilib>:"NT Write Value.vi"("Boolean"=w190, "Name"="CalValueChanged?") -> ()  [unwired: 9 in, 1 out]
              }
            }
          }
          frame "Receive" {
            n126 = property on="Dashboard Tab" class="TabCtl (strict)"() -> ("Pages"=w207:refnum<vi>[])  [unwired: 2 in, 2 out]
            n127 = global read "GlobalDataNames.vi" "stringDataNames"() -> (w201:string)
            n128 = global read "GlobalDataNames.vi" "boolDataNames"() -> (w206:string)
            n129 = global read "GlobalDataNames.vi" "numDataNames"() -> (w203:string)
            n130 = global read "GlobalDataNames.vi" "stringData"() -> (w202:string)
            n131 = global read "GlobalDataNames.vi" "numData"() -> (w204:string)
            n132 = global read "GlobalDataNames.vi" "boolData"() -> (w205:string)
            n133 = Index Array(array=w207, index #1=1 ("index")) -> (element #1=w209:refnum<vi>)  [unwired: 4 in, 4 out]
            n134 = property class="Page"(reference=w209) -> ("ControlsOnPage"=w197:refnum<vi>[])  [unwired: 1 in, 2 out]
            n135 = call-poly <vilib>:"NT Read Value.vi"("Name"=w205) -> ("Boolean Array"=w200:bool[])  [unwired: 9 in, 1 out]
            n136 = call-poly <vilib>:"NT Read Value.vi"("Name"=w206) -> ("String Array"=w199:string[])  [unwired: 9 in, 1 out]
            n137 = call-poly <vilib>:"NT Read Value.vi"("Name"=w204) -> ("Numeric Array"=w195:dbl[])  [unwired: 9 in, 1 out]
            n138 = call-poly <vilib>:"NT Read Value.vi"("Name"=w203) -> ("String Array"=w194:string[])  [unwired: 9 in, 1 out]
            n139 = call-poly <vilib>:"NT Read Value.vi"("Name"=w202) -> ("String Array"=w198:string[])  [unwired: 9 in, 1 out]
            n140 = call-poly <vilib>:"NT Read Value.vi"("Name"=w201) -> ("String Array"=w196:string[])  [unwired: 9 in, 1 out]
            n141 = call "NTToDash.vim"("Controls on Page[]"=w197, "Names Array"=w199, "Data Array"=w200) -> ()  [unwired: 1 in]
            n142 = call "NTToDash.vim"("Controls on Page[]"=w197, "Names Array"=w194, "Data Array"=w195) -> ()  [unwired: 1 in]
            n143 = call "NTToDash.vim"("Controls on Page[]"=w197, "Names Array"=w196, "Data Array"=w198) -> ()  [unwired: 1 in]
          }
        }
      }
    }
  }
  n144 = Bundle("Camera Image"=w54, "Dashboard Tab"=w53, "Background"=w49, "Rec Mode"=w42, "Test Slider"=w41, "On/Off"=w40, "Test Ring"=w39, "Rev/Fwd"=w38, "Test Name"=w44, "Motor"=w43, "Progress"=w37, "CheckList"=w47, "Tree"=w46, "Test Tree"=w45, "Command Params"=w32, "Command Selection"=w29, "Execute Command"=w31, "Cmd Status"=w25, "Camera Settings"=w21, "Camera Name"=w20, "Camera Perf"=w19, "Camera Settings Right"=w9, "Camera Name Right"=w8, "Camera Image Right"=w7) -> (w48:T19)  [unwired: 1 in]
  n145 = call "Handle Camera Configuration.vi"("CameraNameRef"=w22, "Display Name"=w2, "ClusterRef"=w23) -> ()  [unwired: 9 in]
  n146 = while {
    tunnel: w74 -> [w223]
    tunnel: w73 -> [_]
    tunnel: w4 -> [w216]
    tunnel: w2 -> [w213]
    stop <- FALSE stop-if-true
    # "Optionally read the DB image,\nlog, or retrieve images from a\nlogged match"
    n147 = local read "NT Connection"() -> (w217:bool)
    n148 = local read "Rec Mode"() -> (w220:enum32{"Stop", "Record", "Playback"})
    n149 = local read "Right Camera Perf"() -> (w211:cluster{"Bandwidth (Mbps)":dbl, "FPS":dbl})
    n150 = Bundle("Camera Name"="Camera Name", w213, "Saved DB Images Info"=w216) -> (w215:T21)  [unwired: 1 in]
    n151 = control-ref of="Camera Perf"() -> (w210:refnum<vi>)
    n152 = call <vilib>:"WPI_CameraRead MJPG for Dashboard_2.vi"("Camera Settings"="Camera Settings", "Rec Mode"=w220, "NT Connection"=w217, "Capture Info"=w215, "Image in"=w223) -> ("perf info"=w212:cluster{"Bandwidth (Mbps)":dbl, "fps":dbl}, "Active"=w221:bool, "Image\\ out"=w222:T4)  [unwired: 4 in]
    n153 = case shown="True" w221 {
      tunnel: w222 -> [w226 w229]
      tunnel: [w226 w228] -> w218
      frame False {
        # "Sleep for 500ms"
        n154 = property on="Camera Image" class="ImageControl"("ROI"=T20 {"Global Rectangle"=[], "Contours"=[]}) -> ()  [unwired: 2 in, 2 out]
        n155 = Wait Until Next ms Multiple(millisecond multiple=u32 500) -> ()  [unwired: 1 out]
      }
      frame True {
        # "Here is where you would annotate,\npossibly process, and display the image"
        # "Update Mbps LED"
        n156 = call "IMAQ Clear Overlay"("Image"=w229) -> ("error out"=w230:errorcluster, "Image Out"=w228:T4)  [unwired: 2 in, 7 out]
        n157 = Unbundle By Name(w230) -> ("status"=w231:bool)
        n158 = property on="Image Message" class="Str"("Visible"=w231) -> ()  [unwired: 2 in, 2 out]
      }
    }
    "Camera Image" <- w218
    n159 = call <vilib>:"WPI_DashboardFormatPerf.vi"("Right Camera Perf"=w211, "Performance"=w212, "String in"=w210) -> ()  [unwired: 9 in]
  }
  n160 = call "Handle Camera Configuration.vi"("CameraNameRef"=w10, "Display Name"=w3, "ClusterRef"=w11) -> ()  [unwired: 9 in]
  n161 = while {
    tunnel: w13 -> [w246]
    tunnel: w12 -> [_]
    tunnel: [w241] -> _
    tunnel: w4 -> [w237]
    tunnel: w3 -> [w234]
    i -> [w241]
    stop <- FALSE stop-if-true
    n162 = local read "NT Connection"() -> (w238:bool)
    n163 = local read "Rec Mode"() -> (w245:enum32{"Stop", "Record", "Playback"})
    n164 = Bundle("Camera Name Right"="Camera Name Right", w234, "Saved DB Images Info"=w237) -> (w236:T22)  [unwired: 1 in]
    n165 = call <vilib>:"WPI_CameraRead MJPG for Dashboard_2.vi"("Camera Settings"="Camera Settings Right", "Rec Mode"=w245, "NT Connection"=w238, "Capture Info"=w236, "Image in"=w246) -> ("perf info"=w232:cluster{"Bandwidth (Mbps)":dbl, "fps":dbl}, "Active"=w240:bool, "Image\\ out"=w243:T4)  [unwired: 4 in]
    n166 = case shown="True" w240 {
      tunnel: w243 -> [w248 w251]
      tunnel: [w248 w251] -> w239
      tunnel: [_ w250] -> w233
      tunnel: w232 -> [_ w250]
      frame False {
        n167 = Wait Until Next ms Multiple(millisecond multiple=u32 500) -> ()  [unwired: 1 out]
        n168 = property on="Camera Image Right" class="ImageControl"("ROI"=T20 {"Global Rectangle"=[], "Contours"=[]}) -> ()  [unwired: 2 in, 2 out]
      }
      frame True {
      }
    }
    "Camera Image Right" <- w239
    "Right Camera Perf" <- w233
  }
  n169 = register-events(refnum<vi> refnum, w26) -> (reference out=w63:refnum<event-registration>, error out=w62:errorcluster)  [unwired: 2 in]
  n170 = call "Initialize Camera and CheckList.vi"("ListBox in"=w47) -> ()  [unwired: 11 in]
  n171 = disable-structure shown="Disabled" {
    disable-tunnel: w58 -> [w255 _]
    disable-tunnel: w50 -> [w254 _]
    disable-tunnel: w48 -> [w253 _]
    disable-tunnel: w34 -> [w252 _]
    frame Disabled {
      n172 = call "Adjust Dashboard Window.vi"("Sizing Refnums"=w253, "Size Constraints"=w254, "VI"=w255, "WIn Mode"=w252) -> ()  [unwired: 8 in]
    }
    frame Enabled {
    }
  }
  n173 = while {
    tunnel: w55 -> [w267]
    tunnel: w35 -> [w265]
    tunnel: [w263] -> _
    tunnel: u32 1000 ("milliseconds to wait") -> [w262]
    tunnel: w26 -> [w256]
    i -> [w263]
    stop <- FALSE stop-if-true
    n174 = local read "Rec Mode"() -> (w258:enum32{"Stop", "Record", "Playback"})
    n175 = Wait on Notification(notifier=w265, timeout in ms (-1)=w262) -> (notification=w264:string, timed out?=w260:bool)  [unwired: 2 in, 2 out]
    n176 = Equal?(x=w258, y=u16 2 ("Rec Mode")) -> (x = y?=w259:bool)
    n177 = Compound Arithmetic op=OR(invert w260, w259) -> (w261:bool)
    n178 = case shown="True" w261 {
      tunnel: w267 -> [_ w270]
      tunnel: w264 -> [_ w269]
      tunnel: w256 -> [_ w268]
      frame False {
      }
      frame True {
        n179 = call <vilib>:"Bind Controls to SmartDashboard.vi"("RPC ref"=w268, "Bound Control Refs"=w270, "Server IP Address"=w269) -> ()  [unwired: 9 in]
      }
    }
  }
  n180 = vi-ref "Playback Controls.vi"() -> (w64:refnum<vi>)
  n181 = property class="VI"() -> ("Panel"=w66:refnum<vi>)  [unwired: 2 in, 2 out]
  n182 = property class="Pnl"(reference=w66) -> ("Panes[]"=w67:refnum<vi>[])  [unwired: 1 in, 2 out]
  n183 = Index Array(array=w67) -> (element=w65:refnum<vi>)  [unwired: 1 in]
  n184 = control-ref of="Test Tree"() -> (w68:refnum<vi>)
  n185 = while {
    tunnel: [w280] -> _
    tunnel: w68 -> [w279]
    tunnel: w64 -> [w278]
    tunnel: w63 -> [w277]
    tunnel: w62 -> [_]
    tunnel: w58 -> [w276]
    tunnel: w26 -> [w275]
    tunnel: w24 -> [w274]
    shift-right: [w273] -> _
    shift-left: _ -> [w272]
    tunnel: w18 -> [w271]
    i -> [w280]
    stop <- FALSE stop-if-true
    n186 = event shown="[0] Timeout" {
      selector: w277 -> [_ _ _ _ _ _ _ _ _ _ _ _ _ _ _ _ _ _ _ _ _]
      dyn-events: [_ _ _ _ _ _ _ _ _ _ _ _ _ _ _ _ w540 _ _ _ _] -> _
      timeout: u32 60 ("milliseconds to wait") -> [_ _ _ _ _ _ _ _ _ _ _ _ _ _ _ _ _ _ _ _ _]
      tunnel: w279 -> [w292 _ _ _ _ _ _ _ _ _ _ _ _ _ _ _ _ _ _ _ _]
      tunnel: "Test Tree" -> [_ _ _ _ _ _ _ _ _ _ _ w507 w515 w517 w521 w529 _ _ _ _ _]
      tunnel: w278 -> [_ _ _ _ _ _ _ _ _ _ _ _ _ _ _ _ w542 _ w560 _ _]
      tunnel: w276 -> [_ _ _ _ _ _ _ _ _ _ _ _ _ _ _ _ w538 _ _ _ _]
      tunnel: w275 -> [_ _ _ _ _ _ _ _ _ _ _ _ _ _ _ _ w536 _ _ _ _]
      tunnel: w274 -> [w287 _ _ _ _ _ w458 _ _ _ _ _ _ _ _ _ _ _ _ _ _]
      tunnel: [w286 w335 w437 w442 w451 w455 w456 w465 w475 w482 w494 w506 w513 w516 w520 w528 w535 w555 w557 w561 w574] -> w273
      tunnel: w272 -> [w286 w335 w437 w442 w451 w455 w456 _ _ w482 w494 w506 w513 w516 w520 w528 w535 w555 w557 w561 w574]
      tunnel: w271 -> [w284 _ _ _ _ _ _ _ _ _ _ _ _ _ _ _ _ _ _ _ _]
      event Timeout {
        n187 = event-data() -> ()  [unwired: 1 in, 1 out]
        n188 = local read "Mode"() -> (w289:T6)
        n189 = case shown="\"Test\"" "Dashboard Tab" {
          tunnel: w292 -> [_ _ w308 _ _]
          tunnel: "TestMode/Automatic/" ("Name Pattern") -> [_ _ w307 _ _]
          tunnel: T23 [{"Operation"=enum."Clear", "Color Box"=14013909}, {"Operation"=enum."Clear", "Color Box"=14013909}, {"Operation"=enum."Clear", "Color Box"=14013909}, {"Operation"=enum."Clear", "Color Box"=14013909}, {"Operation"=enum."Update", "Color Box"=14013909}, {"Operation"=enum."Update", "Color Box"=16777215}, {"Operation"=enum."Clear", "Color Box"=14013909}, {"Operation"=enum."Clear", "Color Box"=14013909}, {"Operation"=enum."Clear", "Color Box"=14013909}] -> [_ _ w300 _ w328]
          tunnel: w289 -> [_ _ w299 _ w327]
          tunnel: u32[] [15790320, 15790320, 15790320, 15790320, 16777215, 16777215, 15790320, 15790320, 15790320] -> [_ _ _ _ w333]
          tunnel: w287 -> [_ _ _ _ w321]
          tunnel: w284 -> [_ w294 _ _ _]
          frame "Custom", Default {
          }
          frame "Basic" {
            n190 = call <vilib>:"WPI_DashboardUpdateNames.vi"("Controls on Tab"=w294) -> ()  [unwired: 11 in]
          }
          frame "Test" {
            w306 = -2 ("Active Item:Row Number")
            n191 = Index Array(array=w300, index=w299) -> (element=w301:T26)
            n192 = Unbundle(w301) -> ("Operation"=w302:enum16{"Update", "Clear"}, "Color Box"=w303:u32)
            n193 = call <vilib>:"NT Read String.vi"("Name"="TestMode/TestName") -> ("String"=w297:string)  [unwired: 9 in, 1 out]
            n194 = call <vilib>:"NT Read and Format Entries as Tree.vi"("Operation"=w302, "Name Pattern"=w307, "Tree Refnum"=w308) -> ()  [unwired: 7 in, 2 out]
            n195 = case shown="\"\"" w297 {
              tunnel: "TestMode/TestProgress" ("Name") -> [w310 _]
              tunnel: "TestMode/TestProgressText" ("Name") -> [w309 _]
              frame Default {
                n196 = call <vilib>:"NT Read Number.vi"("Name"=w310) -> ("Numeric"=w311:dbl)  [unwired: 9 in, 1 out]
                n197 = call <vilib>:"NT Read String.vi"("Name"=w309) -> ("String"=w312:string)  [unwired: 9 in, 1 out]
                n198 = Bundle("Numeric"=w311, "String"=w312) -> (→"Progress":cluster{"Numeric":dbl, "String":string})  [unwired: 1 in]
              }
              frame "" {
                n199 = property on="Progress" class="Clust (strict)"("Visible"=FALSE) -> ()  [unwired: 2 in, 2 out]
                n200 = local write "Test Name"(u16 0) -> ()
              }
            }
            n201 = property on="Test Tree" class="Tree (strict)"("Active Item Row Number"=w306, "ActiveColNum"=w306, "CellBG"=w303, "Active Item Row Number"=-1 ("Active Item:Row Number"), "CellBG"=u32 5789784 ("Color Box")) -> ()  [unwired: 2 in, 2 out]
          }
          frame "Variables" {
            w318 = string[] ["CameraPublisher", "Usage", "DB"]  # Items to initially close
            n202 = First Call?() -> (First Call?: T/F=w319:bool)
            n203 = control-ref of="Tree"() -> (w320:refnum<vi>)
            n204 = Select(t=w318, s=w319, f=string[] []) -> (s? t:f=w316:string[])
            n205 = call <vilib>:"NT Read and Format Entries as Tree.vi"("Tags to  Close"=w316, "Tree Refnum"=w320) -> ()  [unwired: 8 in, 2 out]
          }
          frame "Commands" {
            w329 = u32 5789784 ("Color Box")
            w330 = T27 {"Row"=-1, "Column"=-2} ("Active Cell:Active Cell")
            w332 = T27 {"Row"=-2, "Column"=-2} ("Active Cell:Active Cell")
            n206 = Index Array(array=w333, index=w327) -> (element=w331:u32)
            n207 = Index Array(array=w328, index=w327) -> (element=w326:T26)
            n208 = Unbundle(w326) -> ("Operation"=w325:enum16{"Update", "Clear"})  [unwired: 1 out]
            n209 = local read "Command Selection"() -> (w324:i32)
            n210 = property on="Command Selection" class="MCListbox (strict)"("ActiveCell"=w332, "CellBG"=w331, "ActiveCell"=w330, "CellBG"=w329) -> ()  [unwired: 2 in, 2 out]
            n211 = call <vilib>:"WPI_DashboardUpdate RPC Info.vi"("Operation"=w325) -> ("update"=w323:bool, "commands"=w322:string[][])  [unwired: 9 in]
            n212 = property on="Command Selection" class="MCListbox (strict)"("ItemNames"=w322) -> ()  [unwired: 2 in, 2 out]
            n213 = property on="Command Params" class="Tbl (strict)"("Active Cell"=w332, "Cell BG Color"=w331, "Active Cell"=w330, "Cell BG Color"=w329) -> ()  [unwired: 2 in, 2 out]
            n214 = call <vilib>:"WPI_DashboardUpdate Command Params.vi"("Update"=w323, "NewVal"=w324, "Commands"=w322, "Param Tbl"=w321) -> ()  [unwired: 7 in, 1 out]
          }
        }
        n215 = call <vilib>:"Connextion Info.vi"() -> ("Connected"=→"NT Connection":bool)  [unwired: 10 in, 1 out]
      }
      event "Test Tree": Value Change {
        # "Show appropriate\ncontrols"
        n216 = event-data() -> ("CtlRef"=w338:refnum<vi>, "NewVal"=w336:string)  [unwired: 1 in]
        n217 = call <vilib>:"WPI_UtilitiesGetTreeIOName.vi"("NewVal"=w336, "TreeControl in"=w338) -> ("I/O Name"=w339:string)  [unwired: 9 in]
        n218 = case shown="\"Camera\"" w339 {
          selector: w339 -> [_ w346 _ w368 w377 _]
          tunnel: w336 -> [_ _ w365 w367 _ w384]
          tunnel: cluster{string[]}[] [{["640x480", "320x240", "160x120"]}, {["Auto", "Fixed indoor", "Fixed outdoor 1", "Fixed outdoor 2", "Fixed fluorescent 1", "Fixed fluorescent 2", "Hold current"]}, {["Auto", "Flicker-free 50 Hz", "Flicker-free 60 Hz", "Hold current"]}, {["None", "Prioritize frame rate", "Prioritize image quality"]}, {["Monochrome", "Color"]}] -> [_ _ _ _ _ w383]
          frame Default {
            w341 = FALSE ("Visible")
            w340 = FALSE ("Visible")
            n219 = property on="Motor" class="Clust (strict)"("Visible"=w340) -> ()  [unwired: 2 in, 2 out]
            n220 = property on="Test Ring" class="Ring (strict)"("Visible"=w340) -> ()  [unwired: 2 in, 2 out]
            n221 = property on="Rev/Fwd" class="Clust (strict)"("Visible"=w341) -> ()  [unwired: 2 in, 2 out]
            n222 = property on="On/Off" class="Bool (strict)"("Visible"=w341) -> ()  [unwired: 2 in, 2 out]
            n223 = property on="Test Slider" class="Slide (strict)"("Visible"=w341) -> ()  [unwired: 2 in, 2 out]
          }
          frame "Analog Out", "Motor", "PWM" {
            w347 = FALSE ("Visible")
            n224 = case shown="\"Analog Out\"" w346 {
              tunnel: [1.0 ("Value") -1.0 ("Value") 0.0 ("Value")] -> w345
              tunnel: [255.0 ("Value") 1.0 ("Value") 5.0 ("Value")] -> w344
              tunnel: [128.0 ("Value") 0.0 ("Value") 0.0 ("Value")] -> w343
              tunnel: [64.0 ("Value") 0.5 ("Value") 1.0 ("Value")] -> w342
              frame "PWM" {
              }
              frame "Motor", Default {
              }
              frame "Analog Out" {
              }
            }
            n225 = property on="Motor" class="Clust (strict)"("Visible"=TRUE) -> ()  [unwired: 2 in, 2 out]
            n226 = property on="Value" class="Slide (strict)"("Value"=w343, "Scale.Minimum"=w345, "Scale.Maximum"=w344, "Scale.Increment"=w342) -> ()  [unwired: 2 in, 2 out]
            n227 = property on="On/Off" class="Bool (strict)"("Visible"=w347) -> ()  [unwired: 2 in, 2 out]
            n228 = property on="Test Slider" class="Slide (strict)"("Visible"=w347) -> ()  [unwired: 2 in, 2 out]
            n229 = property on="Test Ring" class="Ring (strict)"("Visible"=w347) -> ()  [unwired: 2 in, 2 out]
            n230 = property on="Rev/Fwd" class="Clust (strict)"("Visible"=w347) -> ()  [unwired: 2 in, 2 out]
          }
          frame "Servo" {
            w363 = FALSE ("Visible")
            n231 = call <vilib>:"NT Read Number.vi"("Name"=w365) -> ("Numeric"=w364:dbl)  [unwired: 9 in, 1 out]
            n232 = property on="Test Slider" class="Slide (strict)"("Visible"=TRUE, "Scale.Maximum"=170.0 ("Scale.Range:Maximum")) -> ()  [unwired: 2 in, 2 out]
            n233 = local write "Test Slider"(w364) -> ()
            n234 = property on="Motor" class="Clust (strict)"("Visible"=w363) -> ()  [unwired: 2 in, 2 out]
            n235 = property on="Rev/Fwd" class="Clust (strict)"("Visible"=w363) -> ()  [unwired: 2 in, 2 out]
            n236 = property on="On/Off" class="Bool (strict)"("Visible"=w363) -> ()  [unwired: 2 in, 2 out]
            n237 = property on="Test Ring" class="Ring (strict)"("Visible"=w363) -> ()  [unwired: 2 in, 2 out]
          }
          frame "Relay", "Solenoid" {
            w366 = FALSE ("Visible")
            n238 = property on="Motor" class="Clust (strict)"("Visible"=w366) -> ()  [unwired: 2 in, 2 out]
            n239 = property on="Test Slider" class="Slide (strict)"("Visible"=w366) -> ()  [unwired: 2 in, 2 out]
            n240 = Search and Replace String(input string=w367, search string="/Value  **", replace string="/Direction") -> (result string=w373:string)  [unwired: 5 in, 3 out]
            n241 = property on="Test Ring" class="Ring (strict)"("Visible"=w366) -> ()  [unwired: 2 in, 2 out]
            n242 = call <vilib>:"NT Read String.vi"("Name"=w373) -> ("String"=w371:string)  [unwired: 9 in, 1 out]
            n243 = Equal?(x="Both directions", y=w371) -> (x = y?=w369:bool)
            n244 = Not(x=w369) -> (.not. x?=w370:bool)
            n245 = property on="Rev/Fwd" class="Clust (strict)"("Visible"=w369) -> ()  [unwired: 2 in, 2 out]
            n246 = property on="On/Off" class="Bool (strict)"("Visible"=w370, "Caption.Text"=w368) -> ()  [unwired: 2 in, 2 out]
          }
          frame "Compressor", "Digital Out" {
            w376 = FALSE ("Visible")
            # "Get direction and finish"
            n247 = property on="Motor" class="Clust (strict)"("Visible"=w376) -> ()  [unwired: 2 in, 2 out]
            n248 = property on="Test Slider" class="Slide (strict)"("Visible"=w376) -> ()  [unwired: 2 in, 2 out]
            n249 = property on="Test Ring" class="Ring (strict)"("Visible"=w376) -> ()  [unwired: 2 in, 2 out]
            n250 = property on="On/Off" class="Bool (strict)"("Visible"=TRUE, "Caption.Text"=w377) -> ()  [unwired: 2 in, 2 out]
            n251 = property on="Rev/Fwd" class="Clust (strict)"("Visible"=FALSE) -> ()  [unwired: 2 in, 2 out]
          }
          frame "Camera" {
            n252 = call <vilib>:"Get Last Path Segment.vi"("String in"=w384) -> ("String out"=w385:string)  [unwired: 10 in]
            n253 = property on="On/Off" class="Bool (strict)"("Visible"=FALSE) -> ()  [unwired: 2 in, 2 out]
            n254 = property on="Motor" class="Clust (strict)"("Visible"=FALSE) -> ()  [unwired: 2 in, 2 out]
            n255 = property on="Rev/Fwd" class="Clust (strict)"("Visible"=FALSE) -> ()  [unwired: 2 in, 2 out]
            n256 = case shown="\"White Balance  **\"" w385 {
              tunnel: w384 -> [w391 w400 w409 w418 w427 _ w433]
              tunnel: w383 -> [w389 w397 w406 w415 w424 _ _]
              frame "Size  **" {
                n257 = Index Array(array=w389) -> (element=w388:cluster{string[]})  [unwired: 1 in]
                n258 = call <vilib>:"NT Read String.vi"("Name"=w391) -> ("String"=w390:string)  [unwired: 9 in, 1 out]
                n259 = Unbundle(w388) -> (w386:string[])
                n260 = Match First String(2:w386, 3:w390) -> (0:w387:i32)  [unwired: 1 out]
                n261 = property on="Test Ring" class="Ring (strict)"("Value"=w387, "Strings []"=w386) -> ()  [unwired: 2 in, 2 out]
                n262 = property on="Test Ring" class="Ring (strict)"("Visible"=TRUE) -> ()  [unwired: 2 in, 2 out]
                n263 = property on="Test Slider" class="Slide (strict)"("Visible"=FALSE) -> ()  [unwired: 2 in, 2 out]
              }
              frame "White Balance  **" {
                n264 = Index Array(array=w397, index=1) -> (element=w398:cluster{string[]})
                n265 = call <vilib>:"NT Read String.vi"("Name"=w400) -> ("String"=w399:string)  [unwired: 9 in, 1 out]
                n266 = Unbundle(w398) -> (w395:string[])
                n267 = Match First String(2:w395, 3:w399) -> (0:w394:i32)  [unwired: 1 out]
                n268 = property on="Test Ring" class="Ring (strict)"("Value"=w394, "Strings []"=w395) -> ()  [unwired: 2 in, 2 out]
                n269 = property on="Test Ring" class="Ring (strict)"("Visible"=TRUE) -> ()  [unwired: 2 in, 2 out]
                n270 = property on="Test Slider" class="Slide (strict)"("Visible"=FALSE) -> ()  [unwired: 2 in, 2 out]
              }
              frame "Exposure  **" {
                n271 = Index Array(array=w406, index=2) -> (element=w407:cluster{string[]})
                n272 = call <vilib>:"NT Read String.vi"("Name"=w409) -> ("String"=w408:string)  [unwired: 9 in, 1 out]
                n273 = Unbundle(w407) -> (w403:string[])
                n274 = Match First String(2:w403, 3:w408) -> (0:w404:i32)  [unwired: 1 out]
                n275 = property on="Test Ring" class="Ring (strict)"("Value"=w404, "Strings []"=w403) -> ()  [unwired: 2 in, 2 out]
                n276 = property on="Test Ring" class="Ring (strict)"("Visible"=TRUE) -> ()  [unwired: 2 in, 2 out]
                n277 = property on="Test Slider" class="Slide (strict)"("Visible"=FALSE) -> ()  [unwired: 2 in, 2 out]
              }
              frame "Exposure Priority  **" {
                n278 = Index Array(array=w415, index=3) -> (element=w416:cluster{string[]})
                n279 = call <vilib>:"NT Read String.vi"("Name"=w418) -> ("String"=w417:string)  [unwired: 9 in, 1 out]
                n280 = Unbundle(w416) -> (w412:string[])
                n281 = Match First String(2:w412, 3:w417) -> (0:w413:i32)  [unwired: 1 out]
                n282 = property on="Test Ring" class="Ring (strict)"("Value"=w413, "Strings []"=w412) -> ()  [unwired: 2 in, 2 out]
                n283 = property on="Test Ring" class="Ring (strict)"("Visible"=TRUE) -> ()  [unwired: 2 in, 2 out]
                n284 = property on="Test Slider" class="Slide (strict)"("Visible"=FALSE) -> ()  [unwired: 2 in, 2 out]
              }
              frame "Color Enable  **" {
                n285 = Index Array(array=w424, index=4) -> (element=w425:cluster{string[]})
                n286 = call <vilib>:"NT Read String.vi"("Name"=w427) -> ("String"=w426:string)  [unwired: 9 in, 1 out]
                n287 = Unbundle(w425) -> (w421:string[])
                n288 = Match First String(2:w421, 3:w426) -> (0:w422:i32)  [unwired: 1 out]
                n289 = property on="Test Ring" class="Ring (strict)"("Value"=w422, "Strings []"=w421) -> ()  [unwired: 2 in, 2 out]
                n290 = property on="Test Ring" class="Ring (strict)"("Visible"=TRUE) -> ()  [unwired: 2 in, 2 out]
                n291 = property on="Test Slider" class="Slide (strict)"("Visible"=FALSE) -> ()  [unwired: 2 in, 2 out]
              }
              frame Default {
                n292 = property on="Test Ring" class="Ring (strict)"("Visible"=FALSE) -> ()  [unwired: 2 in, 2 out]
                n293 = property on="Test Slider" class="Slide (strict)"("Visible"=FALSE) -> ()  [unwired: 2 in, 2 out]
              }
              frame "Brightness  **", "Color Level  **", "Compression  **", "FPS  **", "Sharpness  **" {
                n294 = call <vilib>:"NT Read Number.vi"("Name"=w433) -> ("Numeric"=w432:dbl)  [unwired: 9 in, 1 out]
                n295 = local write "Test Slider"(w432) -> ()
                n296 = property on="Test Slider" class="Slide (strict)"("Visible"=TRUE, "Scale.Maximum"=100.0 ("Scale.Range:Maximum")) -> ()  [unwired: 2 in, 2 out]
                n297 = property on="Test Ring" class="Ring (strict)"("Visible"=FALSE) -> ()  [unwired: 2 in, 2 out]
              }
            }
          }
        }
        n298 = property on="Progress" class="Clust (strict)"("Visible"=FALSE) -> ()  [unwired: 2 in, 2 out]
      }
      event "Test Name": Mouse Enter {
        # "Populate the ring with the list of tests"
        n299 = event-data() -> ()  [unwired: 1 in, 1 out]
        n300 = call <vilib>:"NT Read String Array.vi"("Name"="TestMode/TestList") -> ("String Array"=w441:string[])  [unwired: 9 in, 1 out]
        n301 = Build Array (concatenate)("Select the test to run...", w441) -> (w440:string[])
        n302 = property on="Test Name" class="Ring (strict)"("Strings []"=w440) -> ()  [unwired: 2 in, 2 out]
      }
      event "Test Name": Value Change {
        w443 = FALSE ("Visible")
        # "Tell the robot the test name to run"
        n303 = event-data() -> ("NewVal"=w447:u16)  [unwired: 1 in]
        n304 = property on="Test Name" class="Ring (strict)"() -> ("Strings []"=w448:string[])  [unwired: 2 in, 2 out]
        n305 = local write "Progress"(T7 {"Test Progress"=0, "Test Progress Text"=""} ("Progress")) -> ()
        n306 = Index Array(array=w448, index=w447) -> (element=w446:string)
        n307 = call <vilib>:"NT Write String.vi"("String"=w446, "Name"="TestMode/TestName") -> ()  [unwired: 9 in, 1 out]
        n308 = property on="Progress" class="Clust (strict)"("Visible"=TRUE) -> ()  [unwired: 2 in, 2 out]
        n309 = property on="Motor" class="Clust (strict)"("Visible"=w443) -> ()  [unwired: 2 in, 2 out]
        n310 = property on="Test Slider" class="Slide (strict)"("Visible"=w443) -> ()  [unwired: 2 in, 2 out]
        n311 = property on="On/Off" class="Bool (strict)"("Visible"=w443) -> ()  [unwired: 2 in, 2 out]
        n312 = property on="Rev/Fwd" class="Clust (strict)"("Visible"=w443) -> ()  [unwired: 2 in, 2 out]
        n313 = property on="Test Ring" class="Ring (strict)"("Visible"=w443) -> ()  [unwired: 2 in, 2 out]
      }
      event "Select Auto": Mouse Enter {
        # "Populate the combo box with the list of autonomous options"
        n314 = event-data() -> ()  [unwired: 1 in, 1 out]
        n315 = call <vilib>:"NT Read String Array.vi"("Name"="Auto List") -> ("String Array"=w450:string[])  [unwired: 9 in, 1 out]
        n316 = property on="Select Auto" class="CmbBox"("Strings[]"=w450) -> ()  [unwired: 2 in, 2 out]
      }
      event "Select Auto": Value Change {
        # "User modified the Auto Selection. Write to NT variable so robot knows."
        n317 = event-data() -> ("NewVal"=w453:string)  [unwired: 1 in]
        n318 = call <vilib>:"NT Write String.vi"("String"=w453, "Name"="Auto Selector") -> ()  [unwired: 9 in, 1 out]
      }
      event "Command Selection": Value Change {
        # "Get the params and show in table"
        n319 = event-data() -> ("NewVal"=w459:i32)  [unwired: 1 in]
        n320 = property on="Command Selection" class="MCListbox (strict)"() -> ("ItemNames"=w457:string[][])  [unwired: 2 in, 2 out]
        n321 = call <vilib>:"WPI_DashboardUpdate Command Params.vi"("NewVal"=w459, "Commands"=w457, "Param Tbl"=w458) -> ()  [unwired: 8 in, 1 out]
      }
      event "Execute Command": Value Change {
        # "Started one, Unique ID holds\nresponse"
        n322 = event-data() -> ()  [unwired: 1 in, 1 out]
        n323 = property on="Command Selection" class="MCListbox (strict)"() -> ("ItemNames"=w470:string[][])  [unwired: 2 in, 2 out]
        n324 = Index Array(array=w470, index (row)="Command Selection", index (col)=0) -> (element=w468:string)
        n325 = call <vilib>:"Invoke Commands.vi"("Command Params"="Command Params", "Function Name"=w468) -> ("Params"=w464:u8, "Started"=w463:bool)  [unwired: 7 in, 1 out]
        n326 = Array Subset(array="Command Params", length (row)=w464) -> (w465:string[][])  [unwired: 3 in]
        n327 = Select(t="Executing" ("Cmd Status"), s=w463, f="" ("Cmd Status")) -> (s? t:f=→"Cmd Status":string)
      }
      event "Command Selection": Double Click {
        n328 = event-data() -> ("Row"=w478:i32)  [unwired: 1 in]
        n329 = property on="Command Selection" class="MCListbox (strict)"() -> ("ItemNames"=w481:string[][])  [unwired: 2 in, 2 out]
        n330 = local read "Command Params"() -> (w477:string[][])
        n331 = Index Array(array=w481, index (row)=w478, index (col)=0) -> (element=w479:string)
        n332 = call <vilib>:"Invoke Commands.vi"("Command Params"=w477, "Function Name"=w479) -> ("Params"=w476:u8, "Started"=w471:bool)  [unwired: 7 in, 1 out]
        n333 = Array Subset(array=w477, length (row)=w476) -> (w475:string[][])  [unwired: 3 in]
        n334 = Select(t="Executing" ("Cmd Status"), s=w471, f="" ("Cmd Status")) -> (s? t:f=w472:string)
        n335 = local write "Cmd Status"(w472) -> ()
      }
      event "CheckList": Double Click {
        # "Shift clears all"
        # "Update symbols on the listbox"
        n336 = event-data() -> ("PlatMods.Shift"=w483:bool, "Row"=w485:i32)  [unwired: 1 in]
        n337 = case shown="True" w483 {
          tunnel: w485 -> [w489 _]
          tunnel: 1 -> [w488 _]
          frame False {
            n338 = property on="CheckList" class="LstBox (strict)"() -> ("Item Symbols"=w487:i32[])  [unwired: 2 in, 2 out]
            n339 = Replace Array Subset(array=w487, new element=w488, index=w489) -> (w486:i32[])
            n340 = property on="CheckList" class="LstBox (strict)"("Item Symbols"=w486) -> ()  [unwired: 2 in, 2 out]
          }
          frame True {
            w490 = 0 ("Top Row")
            n341 = property on="CheckList" class="LstBox (strict)"() -> ("Number of Rows"=w492:u32)  [unwired: 2 in, 2 out]
            n342 = Initialize Array(0, w492) -> (w491:i32[])
            n343 = property on="CheckList" class="LstBox (strict)"("Top Row"=w490, "Value"=w490, "Item Symbols"=w491) -> ()  [unwired: 2 in, 2 out]
          }
        }
      }
      event "CheckList": Key Down {
        # "Update symbols on the listbox\nLeft and right keys check and uncheck"
        n344 = event-data() -> ("VKey"=w496:T24)  [unwired: 1 in]
        n345 = case shown="\"Left\", \"Right\"" w496 {
          selector: w496 -> [w501 _]
          tunnel: eventvkey."Left" ("VKey") -> [w499 _]
          frame "Left", "Right" {
            n346 = Equal?(x=w499, y=w501) -> (x = y?=w500:bool)
            n347 = Select(t=0, s=w500, f=1) -> (s? t:f=w502:i32)
            n348 = property on="CheckList" class="LstBox (strict)"() -> ("Item Symbols"=w505:i32[])  [unwired: 2 in, 2 out]
            n349 = Replace Array Subset(array=w505, new element=w502, index="CheckList") -> (w504:i32[])
            n350 = property on="CheckList" class="LstBox (strict)"("Item Symbols"=w504) -> ()  [unwired: 2 in, 2 out]
          }
          frame Default {
          }
        }
      }
      event "Motor.Enable": Value Change {
        # "When the test mode otor enable helper is set, update that\ntree row item's value"
        n351 = event-data() -> ("NewVal"=w511:bool)  [unwired: 1 in]
        n352 = Unbundle("Motor") -> ("Value"=w510:dbl)  [unwired: 1 out]
        n353 = Select(t=w510, s=w511, f=0.0) -> (s? t:f=w508:dbl)
        n354 = call <vilib>:"NT Write Number.vi"("Numeric"=w508, "Name"=w507) -> ()  [unwired: 9 in, 1 out]
      }
      event "Test Slider": Value Change {
        # "When the test mode slider helper is set, update that\ntree row item's value"
        n355 = event-data() -> ("NewVal"=w514:dbl)  [unwired: 1 in]
        n356 = call <vilib>:"NT Write Number.vi"("Numeric"=w514, "Name"=w515) -> ()  [unwired: 9 in, 1 out]
      }
      event "On/Off": Value Change {
        # "When the test mode on/off helper value is set, update that\ntree row item's value"
        n357 = event-data() -> ("NewVal"=w519:bool)  [unwired: 1 in]
        n358 = Boolean To (0,1)(Boolean=w519) -> (0, 1=w518:i16)
        n359 = call <vilib>:"NT Write Number.vi"("Numeric"=w518, "Name"=w517) -> ()  [unwired: 9 in, 1 out]
      }
      event "Rev/Fwd": Value Change {
        # "When the test mode helper value for relays is set, update that\ntree row item's value"
        n360 = event-data() -> ("NewVal.Forward"=w527:bool, "NewVal.Reverse"=w526:bool)  [unwired: 1 in]
        n361 = Boolean To (0,1)(Boolean=w527) -> (0, 1=w523:i16)
        n362 = Boolean To (0,1)(Boolean=w526) -> (0, 1=w525:i16)
        n363 = Negate(x=w525) -> (-x=w524:i16)
        n364 = Add(x=w523, y=w524) -> (x+y=w522:i16)
        n365 = call <vilib>:"NT Write Number.vi"("Numeric"=w522, "Name"=w521) -> ()  [unwired: 9 in, 1 out]
      }
      event "Test Ring": Value Change {
        # "When a test mode helper value is selected from the ring,\nset the tree item's variable to the string value"
        n366 = event-data() -> ("NewVal"=w531:u16)  [unwired: 1 in]
        n367 = property on="Test Ring" class="Ring (strict)"() -> ("Strings []"=w532:string[])  [unwired: 2 in, 2 out]
        n368 = Index Array(array=w532, index=w531) -> (element=w530:string)
        n369 = call <vilib>:"NT Write String.vi"("String"=w530, "Name"=w529) -> ()  [unwired: 9 in, 1 out]
      }
      event "Rec Mode": Value Change {
        # "Update globals for recording mode and path to read log from.\nClear when logging and let NetworkTables set path for vision to\nuse."
        n370 = event-data() -> ("NewVal"=w543:enum32{"Stop", "Record", "Playback"})  [unwired: 1 in]
        n371 = global write "WPI_DashboardLogging Global.vi" "Logging Filename"(path "") -> ()
        n372 = global write "WPI_DashboardLogging Global.vi" "Recording"(w543) -> ()
        n373 = case shown="\"Playback\"" w543 {
          tunnel: w542 -> [_ w545 w554]
          tunnel: [_ _ w553] -> w540
          tunnel: [_ _ w552] -> _
          tunnel: w538 -> [_ _ w550]
          tunnel: cluster{i32, i32} {-250, 170} -> [_ _ w549]
          tunnel: [_ _ T25 {"Image Size"=TRUE, "Image Type"=TRUE, "Pixel Value"=TRUE, "ROI Information"=TRUE, "Zoom Factor"=FALSE} ("Image Information Shown:All Elements")] -> w533
          tunnel: [_ _ TRUE ("Zoom Factor")] -> w534
          tunnel: w536 -> [_ _ w546]
          frame Default {
          }
          frame "Stop", "Record" {
            # "Place Window too"
            n374 = invoke class="VI" method="FP.Close"(reference=w545) -> (reference out=w544:refnum<vi>)  [unwired: 2 in, 2 out]
            n375 = invoke class="VI" method="Abort VI"(reference=w544) -> ()  [unwired: 2 in, 3 out]
          }
          frame "Playback" {
            n376 = call "Open Playback Panel.vi"("Offset"=w549, "DB VI Ref"=w550, "Playback in"=w554) -> ("Playback out"=w551:refnum<vi>)  [unwired: 8 in]
            n377 = register-events(w551, w546) -> (reference out=w553:refnum<event-registration>, error out=w552:errorcluster)  [unwired: 2 in]
          }
        }
        n378 = property on="Camera Image Right" class="ImageControl"("Image Information Shown"=w533, "Image Information Visible"=w534) -> ()  [unwired: 2 in, 2 out]
        n379 = property on="Camera Image" class="ImageControl"("Image Information Shown"=w533, "Image Information Visible"=w534) -> ()  [unwired: 2 in, 2 out]
        n380 = call <vilib>:"WPI_DashboardNT Log FieldName Cache.vi"("Operation"=enum16{"Lookup/Add", "Index", "Clear"}."Clear") -> ()  [unwired: 8 in, 3 out]
      }
      event Panel Close {
        w556 = enum32{"Stop", "Record", "Playback"}."Stop" ("Rec Mode")
        # "Playback window has been closed, abort"
        n381 = event-data() -> ()  [unwired: 1 in, 4 out]
        n382 = local write "Rec Mode"(w556) -> ()
        n383 = global write "WPI_DashboardLogging Global.vi" "Recording"(w556) -> ()
      }
      event Panel Close {
        # "Abort playback window and ourself"
        n384 = event-data() -> ()  [unwired: 1 in, 4 out]
        n385 = invoke class="VI" method="FP.Close"(reference=w560) -> (reference out=w559:refnum<vi>)  [unwired: 2 in, 2 out]
        n386 = invoke class="VI" method="Abort VI"(reference=w559) -> (error out=w558:errorcluster)  [unwired: 2 in, 2 out]
        n387 = invoke class="VI" method="Abort VI"(error in=w558) -> ()  [unwired: 2 in, 3 out]
      }
      event User Event {
        n388 = event-data() -> ("IDs"=w567:cluster{"RPC field ID":u16, "Unique ID":u16}, "String"=w566:string)  [unwired: 1 in]
        n389 = Bundle("IDs"=w567, "String"=w566) -> (w565:T11)  [unwired: 1 in]
        n390 = call <vilib>:"Retrieve RPC Response.vi"("RPC Response"=w565) -> ("Output"=w563:string[][])  [unwired: 10 in]
        n391 = Build Array (concatenate)(w561, w563) -> (w562:string[][])
        n392 = local write "Command Params"(w562) -> ()
        n393 = local write "Cmd Status"("" ("Cmd Status")) -> ()
      }
      event "Tree": Double Click {
        n394 = event-data() -> ("PlatMods"=w573:T28, "Tag"=w570:string)  [unwired: 1 in]
        n395 = Unbundle(w573) -> ("Shift"=w572:bool)  [unwired: 4 out]
        n396 = String Subset(string=w570, length (rest)=1 ("length (rest)")) -> (substring=w569:string)  [unwired: 1 in]
        n397 = Not(x=w572) -> (.not. x?=w571:bool)
        n398 = case shown="\"/\"" w569 {
          tunnel: w570 -> [_ w576]
          tunnel: w571 -> [_ w575]
          frame Default {
          }
          frame "/" {
            n399 = call <vilib>:"NT Update Persistence.vi"("Persistence"=w575, "Name"=w576) -> ()  [unwired: 9 in, 1 out]
          }
        }
      }
    }
  }
  n400 = while {
    tunnel: w65 -> [w578]
    i -> [w581]
    stop <- FALSE stop-if-true
    n401 = Wait (ms)(milliseconds to wait=u32 100) -> ()  [unwired: 1 out]
    n402 = case shown="\"Playback\"" "Rec Mode" {
      tunnel: w581 -> [_ _ w596]
      tunnel: [u32 2829099 ("Base Color") u32 11141120 ("Target Color") w585] -> w577
      frame "Stop", Default {
        # "Reset the color, extra updates don't cost much"
      }
      frame "Record" {
      }
      frame "Playback" {
        # "Playback"
        n403 = Quotient & Remainder(x=w596, y=u32 50 ("milliseconds to wait")) -> (x-y*floor(x/y)=w592:u32)  [unwired: 1 out]
        n404 = Divide(x=w592, y=u32 50 ("milliseconds to wait")) -> (x/y=w589:dbl)
        n405 = Multiply(x=6.283185307179586, y=w589) -> (x*y=w594:dbl)
        n406 = Sine(x=w594) -> (sin(x)=w593:dbl)
        n407 = Absolute Value(x=w593) -> (abs(x)=w586:dbl)
        n408 = call "Interpolate RGB Color.vi"("Proportion"=w586, "Target Color"=u32 30976, "Base Color"=u32 2829099) -> ("Result Color"=w585:u32)  [unwired: 8 in]
      }
    }
    n409 = property class="Pane"(reference=w578, "PaneColor"=w577) -> ()  [unwired: 1 in, 2 out]
  }
  n410 = local write "Dashboard Tab"(T2."Calibration" ("Dashboard Tab")) -> ()
  n411 = property on="On/Off" class="Bool (strict)"("Visible"=w36) -> ()  [unwired: 2 in, 2 out]
  n412 = property on="Motor" class="Clust (strict)"("Visible"=w36) -> ()  [unwired: 2 in, 2 out]
  n413 = property on="Progress" class="Clust (strict)"("Visible"=w36) -> ()  [unwired: 2 in, 2 out]
  n414 = property on="Test Ring" class="Ring (strict)"("Visible"=w36) -> ()  [unwired: 2 in, 2 out]
  n415 = property on="Rev/Fwd" class="Clust (strict)"("Visible"=w36) -> ()  [unwired: 2 in, 2 out]
  n416 = local write "Command Selection"(u16 0 ("milliseconds to wait")) -> ()
  n417 = while {
    tunnel: u16 1741 ("timeout ms (25000)") -> [w598]
    stop <- FALSE stop-if-true
    n418 = TCP Create Listener(10:w598) -> (0:w597:errorcluster, 3:w599:refnum<k5>)  [unwired: 4 in, 1 out]
    n419 = case shown="No Error" w597 {
      selector: w597 -> [w601 _]
      tunnel: w599 -> [w602 _]
      frame No Error {
        n420 = while {
          tunnel: w602 -> [w605]
          tunnel: w601 -> [w604]
          stop <- FALSE stop-if-true
          n421 = TCP Wait On Listener(8:w604, 11:w605) -> (0:w606:errorcluster, 4:w607:refnum<k5>)  [unwired: 2 in, 3 out]
          n422 = local write "TCP"(w607) -> ()
          n423 = case shown="No Error" w606 {
            frame No Error {
            }
            frame Error {
              n424 = Wait (ms)(milliseconds to wait=u32 1000) -> ()  [unwired: 1 out]
            }
          }
        }
      }
      frame Error {
        n425 = Wait (ms)(milliseconds to wait=u32 1000) -> ()  [unwired: 1 out]
      }
    }
  }
  n426 = local write "Command Params"(string[][] [] ("Command Params")) -> ()
  n427 = global write "WPI_DashboardLogging Global.vi" "Recording"(w59) -> ()
  n428 = local write "Rec Mode"(w59) -> ()
  n429 = call <vilib>:"NT Write String.vi"("String"="Select Auto", "Name"="Auto Selector") -> ()  [unwired: 9 in, 1 out]
  n430 = disable-structure shown="Disabled" {
    frame Disabled {
      n431 = feedback #2() -> (w614)  [unwired: 1 in]
      n432 = feedback-in #2() -> (w613)
      n433 = for {
        tunnel: w614 -> [w618]
        tunnel: w613 -> [w619] mode=indexing
        tunnel: [w617] -> w612 mode=indexing
        n434 = Not Equal?(x=w619, y=w618) -> (x != y?=w617:bool)
      }
      n435 = Or Array Elements(Boolean array=w612) -> (logical OR=w611:bool)
      n436 = call "NTSend.vi"() -> ()  [unwired: 12 in]
      n437 = case shown="True" w611 {
        tunnel: w613 -> [_ w616]
        tunnel: "Sent_Data" ("Name") -> [_ w615]
        frame False {
        }
        frame True {
          n438 = call-poly <vilib>:"NT Write Value.vi"("String Array"=w616, "Name"=w615) -> ()  [unwired: 9 in, 1 out]
        }
      }
    }
    frame Enabled {
    }
  }
  n439 = disable-structure shown="Disabled" {
    disable-tunnel: _ -> [w620 _]
    frame Disabled {
      n440 = for {
        tunnel: w620 -> [w624] mode=indexing
        tunnel: [w623] -> _ mode=indexing
        tunnel: [w622] -> _ mode=indexing
        tunnel: [w621] -> _ mode=indexing
        i -> [w635]
        n441 = call <vilib>:"Get Type Information.vi"("variant"=w624) -> ("type"=w637:T29)  [unwired: 6 in, 4 out]
        n442 = call <vilib>:"Get Type Information.vi"("variant"=w624) -> ("type"=w629:T29)  [unwired: 6 in, 4 out]
        n443 = call <vilib>:"Get Type Information.vi"("variant"=w624) -> ("type"=w628:T29)  [unwired: 6 in, 4 out]
        n444 = Equal?(x=w637, y=Data_Type."String") -> (x = y?=w634:bool)
        n445 = Equal?(x=w629, y=Data_Type."Boolean") -> (x = y?=w631:bool)
        n446 = Equal?(x=w628, y=Data_Type."Double Float") -> (x = y?=w626:bool)
        n447 = Select(t=w635, s=w634, f=-1) -> (s? t:f=w623:i32)
        n448 = Select(s=w631, f=-1) -> (s? t:f=w622:i32)  [unwired: 1 in]
        n449 = Select(s=w626, f=-1) -> (s? t:f=w621:i32)  [unwired: 1 in]
      }
    }
    frame Enabled {
    }
  }
